vi "Old Mixed Mode Widget.vi"() -> ()   [LabVIEW 2009]
uses:
  lib/Data Access Objects/Metadata/LBCB Filter.ctl
  lib/Apps/App Parameters Actions.ctl
  lib/MixedMode/Mixed Mode Command Action.ctl
  lib/MixedMode/Target Data.ctl
  lib/MixedMode/Ramp Time Tuple.ctl
  lib/MixedMode/Messages/Mixed Mode Command.ctl
  lib/MixedMode/Mixed Mode Cartesian Data.ctl
  lib/MixedMode/Mixed Mode Covergance Status.ctl
  lib/MixedMode/Mixed Mode States.ctl
  lib/MixedMode/Messages/Mixed Mode Status.ctl
  lib/Launcher/NoPanelAppTypes.ctl
  lib/Launcher/Launcher Actions.ctl
  lib/MixedMode/Widget/Accepted or Declined.ctl
  lib/NTCP Client/NTCP Msg Types.ctl
  NTCP library/NTCP Commands.ctl
  NTCP library/NTCP Message.ctl
  lib/NTCP Client/NTCP States.ctl
  lib/NTCP Client/Control Point Suffix.ctl
  lib/MixedMode/Widget/Mixed Mode Widget Requests.ctl
  lib/MixedMode/Widget/MM Widget Parameter Changes.ctl
  lib/MixedMode/Widget/Step DAO Actions.ctl
  lib/MixedMode/Widget/Target.ctl
  NTCP library/Payload.ctl
  lib/MixedMode/Widget/Mixed Mode Widget State.ctl
  lib/MixedMode/Widget/NTCP MM Requests.ctl
  lib/Apps/App Status Actions.ctl
  lib/Data Access Objects/Metadata/LBCB Space.ctl
  lib/Global Data/Cartesian Measurment Actions.ctl
  lib/Data Access Objects/Metadata/LBCB Number.ctl
  lib/Global Data/Name Actions.ctl
  lib/Apps/AppStates.ctl
  lib/Control Loop/Parameter Change States.ctl
  lib/Control Loop/Parameters Changes.ctl
  lib/Apps/GUI Control.ctl
  lib/Data Access Objects/Metadata/Persistant DAO Actions.ctl
  lib/MixedMode/Widget/Mixed Mode State Display.ctl
  lib/MixedMode/Widget/Target Pattern.ctl
panel:
  in  "Cartesian Type":bool caption="CartesianType"
  out "NTCP MM Requests":T1
  in  "Connect Server Flag":bool
  out "Force Limit":bool caption="Force"
  out "Displacement Limit":bool caption="Displacement"
  out "Messages":string
  out "Mixed Mode Status":T2={"LBCB Target"=[], "MixedModeStates"=enum."Idle", "LBCB Convergence"=[], "LBCB Measurements"=[]}
  in  "App Running":bool
  out "Mixed Mode Widget Actions":T8
  out "Mixed Mode Widget Requests":T9
  in  "Stop":bool
  out "Mixed Mode Command":T11
  in  "Cartesian Type Button":bool caption="CartesianType"
  in  "Channel Data Tables":T14(tab)
  out "Cartesian Space Labels L1":string[](array[string])=["Commands (in/rad)", "Displacements (in/rad)", "Forces (lbs/lb*in)"]
  out "Cartesian Labels L1":string[](array[string])=["X", "Y", "Z", "Rx", "Ry", "Rz"]
  out "LBCB 1 Cartesian Space":dbl[][](array[numeric]) caption="LBCB 1"
  out "LBCB 2 Cartesian Space":dbl[][](array[numeric]) caption="LBCB 2"
  out "Cartesian Labels L2":string[](array[string])=["X", "Y", "Z", "Rx", "Ry", "Rz"]
  out "Cartesian Space Labels L2":string[](array[string])=["Commands (in/rad)", "Displacements (in/rad)", "Forces (lbs/lb*in)"]
  out "Actuator Space Labels L2":string[](array[string])=["Commands (in)", "Displacements (in)", "Forces (lbs)", "Integral"]
  out "Actuator Labels L2":string[](array[string])=["X1", "X2", "Y1", "Z1", "Z2", "Z3"]
  out "LBCB 2 Actuator Space":dbl[][](array[numeric]) caption="LBCB 2"
  out "LBCB 1 Actuator Space":dbl[][](array[numeric]) caption="LBCB 1"
  out "Actuator Labels L1":string[](array[string])=["X1", "X2", "Y1", "Z1", "Z2", "Z3"]
  out "Actuator Space Labels L1":string[](array[string])=["Commands (in)", "Displacements (in)", "Forces (lbs)", "Integral"]
  out "External Sensors":cluster{"Name":string, "Value":dbl}[](array[cluster])
  out "Test Statistics":cluster{"Steps":string, "Elapsed \nTime":dbl} {"Elapsed \nTime" format="%<%H:%M:%S>T"}
  in  "Mixed Mode Control Type":enum32{"Manual", "Input File", "NTCP"}(tab)
  in  "Target Pattern":T15
  in  "Apply Pattern":bool
  in  "Pause infile":bool
  in  "Run Infile":bool
  in  "Running":bool
  in  "Reset":bool
  in  "LBCB 1":path
  in  "Load File":bool
  in  "LBCB 2":path
  out "NTCP State":T16
  in  "Connect Server":bool
  in  "Control Point":string="MDL-00-01"
  out "Connected":bool
  in  "Execute":cluster{"Auto":bool, "Start":bool, "Stop":bool}
  in  "Propose":T17
  out "Mixed Mode State Display":T18
  out "Current Values":T19[](array[typedef])
  in  "Ramp Times":cluster{"Displacement":T13, "Force":T13}={"Displacement"={"Ramp"=5.0, "Stab"=4.0, "Hold"=5.0}, "Force"={"Ramp"=5.0, "Stab"=4.0, "Hold"=5.0}}
  in  "Targets":T19[](array[typedef])
  # "Limit\nFaults"
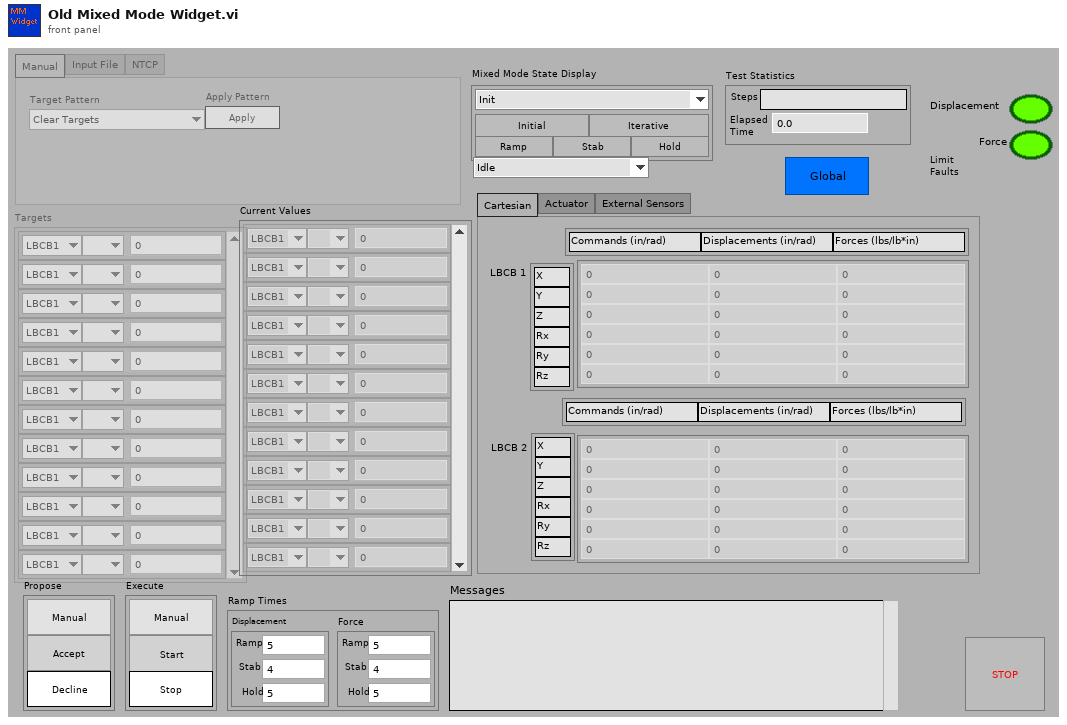
[diagram p1: front panel]
types:
  T1 = typedef "NTCP MM Requests.ctl" = cluster{"Execute Pending":bool, "Propose Pending":bool, "Connected":bool, "Reset":bool}
  T2 = typedef "Mixed Mode Status.ctl" = cluster{"LBCB Target":T3[], "MixedModeStates":T5, "LBCB Convergence":T6[], "LBCB Measurements":T7[]}
  T3 = typedef "Target Data.ctl" = cluster{"Displacements":dbl[], "Command Type":enum16{"<None>", "Displacement", "Force"}[], "Forces":dbl[], "Space":T4}
  T4 = typedef "LBCB Space.ctl" = enum16{"Actuator", "Cartesian"}
  T5 = typedef "Mixed Mode States.ctl" = enum16{"Init", "Wait For DAQ", "Idle", "Start Initial Position", "Initial Position", "Start Initial Ramp", "Run Initial Ramp", "Start Iterative Stage", "Convergence Check", "Update Stiffness Jacobian", "Update Command", "Start Iterative Ramp", "Run Iterative Ramp", "Start Iterative Stabilize", "Iterative Stabilize", "Start Iterative Holding", "Iterative Holding", "Start Stabilize", "Stabilize", "Start Hold", "Holding", "Done", "Aborting", "Exit", "Nop"}
  T6 = typedef "Mixed Mode Covergance Status.ctl" = cluster{"IsConverged":bool[], "Force Errors":dbl[], "MaxForceDiffIndex":i32}
  T7 = typedef "Mixed Mode Cartesian Data.ctl" = cluster{"Displacements":dbl[], "Forces":dbl[]}
  T8 = typedef "Mixed Mode Widget State.ctl" = enum16{"Idle", "Auto Start", "Wait for Start", "Start", "Wait for Hold", "Waiting for Done", "Step Completed", "Limit Fault", "Stop", "Abort", "Clear Targets", "Reset", "Steps Loaded", "Paused", "Steps Available", "Load Step", "Connected", "Disconnecting", "Wait for Proposal", "Auto Accept", "Wait for Accept", "Accept", "Decline", "Wait for Execute", "Unknown", "Exit"}
  T9 = typedef "Mixed Mode Widget Requests.ctl" = cluster{"Start Requested":bool, "Targets Updated":bool, "Targets Cleared":bool, "Stop Requested":bool, "Auto-Start Enabled":bool, "Auto-Accept Enabled":bool, "Accepted or Declined":T10, "Running":bool, "File Loaded":bool, "Reset":bool, "Exit Requested":bool}
  T10 = typedef "Accepted or Declined.ctl" = enum16{"No Decision Yet", "Accepted", "Declined"}
  T11 = typedef "Mixed Mode Command.ctl" = cluster{"Command":T12, "Ramp Times":cluster{"Initial":T13, "Iterative":T13}, "LBCB1":T3, "LBCB2":T3}
  T12 = typedef "Mixed Mode Command Action.ctl" = enum16{"Start Command", "Stop", "Exit", "No Op", "Start Acquisition", "Measure Initial Position"}
  T13 = typedef "Ramp Time Tuple.ctl" = cluster{"Ramp":dbl, "Stab":dbl, "Hold":dbl}
  T14 = enum32{"Cartesian", "Actuator", "External Sensors"}
  T15 = typedef "Target Pattern.ctl" = enum16{"Clear Targets", "Reset Targets to Zero", "Displacements Only", "Rotations Only", "Displacements & Rotations"}
  T16 = typedef "NTCP States.ctl" = enum16{"Init", "Disconnected", "Start Server", "Connect to Server", "Listening", "Parse Message", "Proposed", "Execute", "Get Control Point", "Shutdown Server"}
  T17 = cluster{"Auto":bool, "Accept":bool, "Decline":bool}
  T18 = typedef "Mixed Mode State Display.ctl" = cluster{"MixedModeStates":T5, "Initial":bool, "Iterative":bool, "Ramp":bool, "Stab":bool, "Hold":bool}
  T19 = typedef "Target.ctl" = cluster{"LBCB Number":T20, "DOF Vectors":enum16{" ", "Dx", "Dy", "Dz", "Rx", "Ry", "Rz", "Fx", "Fy", "Fz", "Mx", "My", "Mz"}, "Amount":dbl}
  T20 = typedef "LBCB Number.ctl" = enum16{"LBCB1", "LBCB2"}
  T21 = typedef "GUI Control.ctl" = cluster{"Command":T22, "LBCB Number":enum16{"LBCB1", "LBCB2"}}
  T22 = typedef "MM Widget Parameter Changes.ctl" = enum16{"Start", "Stop All", "Cartesian Type Changed", "Control Enabled", "Control Disabled"}
  T23 = typedef "Parameters Changes.ctl" = cluster{"Change State":T24, "LBCB Number":T20}
  T24 = typedef "Parameter Change States.ctl" = enum16{"Mixed Mode", "Control Loop", "Limits", "Application", "Stiffness Jacobian", "Start DAQ", "Auto-Balancing", "Set Command", "Enable Control", "Disable Control", "Stop Application"}
  T25 = typedef "Name Actions.ctl" = enum16{"Init", "Get Names", "Get Index"}
  T26 = typedef "LBCB Filter.ctl" = enum16{"LBCB 1", "LBCB 2", "Both"}
  T27 = typedef "NTCP Message.ctl" = cluster{"NTCP commands":T28, "Transaction ID":string, "Control Point":string, "Payload":T29[]}
  T28 = typedef "NTCP Commands.ctl" = enum16{"propose", "execute", "cancel", "set-parameter", "get-parameter", "open-session", "close-session", "get-control-point", "Unknown", "stop"}
  T29 = typedef "Payload.ctl" = cluster{"Content":string, "Control Point Suffix":T30}
  T30 = typedef "Control Point Suffix.ctl" = enum16{"LBCB1", "LBCB2", "ExternalSensors"}
  T31 = typedef "Launcher Actions.ctl" = enum16{"Launch", "Stop All", "Stop", "Kill", "Running?", "Init"}
  T32 = typedef "NoPanelAppTypes.ctl" = enum16{"NTCP Socket", "Data Archiving", "DAQ Link", "Control Loops", "Autobalance Monitor", "Mixed Mode Monitor", "Cart Plot", "Act Plot", "Cmd Disp Diffs"}
  T33 = typedef "App Status Actions.ctl" = enum16{"Init", "Get Status", "Running", "Control", "Autobalanced", "Data Acquisition", "Set App State", "DAQ Started", "Set LBCB State", "Set All", "Set Cont Logging", "Set Step Logging", "Set MM Logging", "Set Volt Logging", "Set Cart Type", "Set DAQ Link", "Set NTCP Link"}
  T34 = typedef "Step DAO Actions.ctl" = enum16{"Init", "Set", "Get", "Reset Count"}
  T35 = typedef "App Status.ctl" = cluster{"Running":bool, "Controlling L2":bool, "Autobalance L2":bool, "Data Acquisition":bool, " App State":T36, "DAQ Started":bool, "LBCB 1 State":T37, "LBCB 2 State":T37, "Controlling L1":bool, "Autobalance L1":bool, "Cartesian Type":bool, "Continuous Logging":bool, "Step Logging":bool, "Voltage Logging":bool, "Mixed Mode Logging":bool, "DAQ Link":bool, "NTCP Link ":bool}
  T36 = typedef "AppStates.ctl" = enum16{"Starting OM", "Initializing Displays", "Setting up Archiving", "Setting Up DAQ Channels", "Start DAQ", "DAQ Starting", "Controlling LBCBs", "Stopping OM"}
  T37 = typedef "Lbcb Control Loop States.ctl" = enum16{"Idle", "Start Selected", "Load Last Command", "Start Autobalancing", "Autobalancing", "Control Loop Initialized", "Control Enabled"}
  T38 = typedef "App Parameters Actions.ctl" = enum16{"Init", "Get", "Set"}
  T39 = typedef "Persistant DAO Actions.ctl" = enum16{"Init", "Get", "Set", "Load", "Save"}
  T40 = typedef "App Parameters.ctl" = cluster{"Monitor Loop":T41, "Ramp Time":T41, "Log Loop":T41, "TCP to DAQ":T41, "Logging Directory":path, "Log File Size (MBytes)":i64, "Volt Logging Loop":T41}
  T41 = typedef "Timing Parameters.ctl" = cluster{"Interval":dbl, "Rate ":dbl}
  T42 = typedef "Ramp Time Input.ctl" = cluster{"Directional":T43, "Iterative":T43}
  T43 = typedef "Ramp Control.ctl" = cluster{"Ramp":dbl, "Stabilize":dbl, "Hold":dbl}
  T44 = typedef "Mixed Mode Widget Button States.ctl" = cluster{"Auto-Start Enabled":bool, "Auto-Accept Enabled":bool, "Exit Requested":bool, "Mixed Mode Control Type":T45, "Input File Loaded":bool, "Input File Running":bool}
  T45 = typedef "Mixed Mode Control Type.ctl" = enum32{"Manual", "Input File", "NTCP"}
  T46 = typedef "Widget Changed.ctl" = cluster{"Running Changed":bool, "Apply Pattern Changed":bool, "Propose Changed":bool, "Execute Changed":bool, "Widget Requests Changed":bool}
  T47 = typedef "NTCP Msg Types.ctl" = enum16{"Control Point", "Step Done", "Propose Accepted", "Propose Not Accepted", "Propose Declined", "Propose Response", "Execute Done"}
  T48 = typedef "Cartesian Measurment Actions.ctl" = enum16{"Set Data", "Get", "Init", "Set Offsets"}
  T49 = typedef "Cartesian Data Type.ctl" = cluster{"Displacements":dbl[], "Forces":dbl[], "Displacement Commands":dbl[]}
  T50 = typedef "Propose Command.ctl" = cluster{"Control Type":i32[], "Value":dbl[]}
  T51 = typedef "Mixed Mode Blinkies.ctl" = cluster{"Blink Accept":bool, "Blink Start":bool, "Targets Updated":bool, "Disconnect":bool}
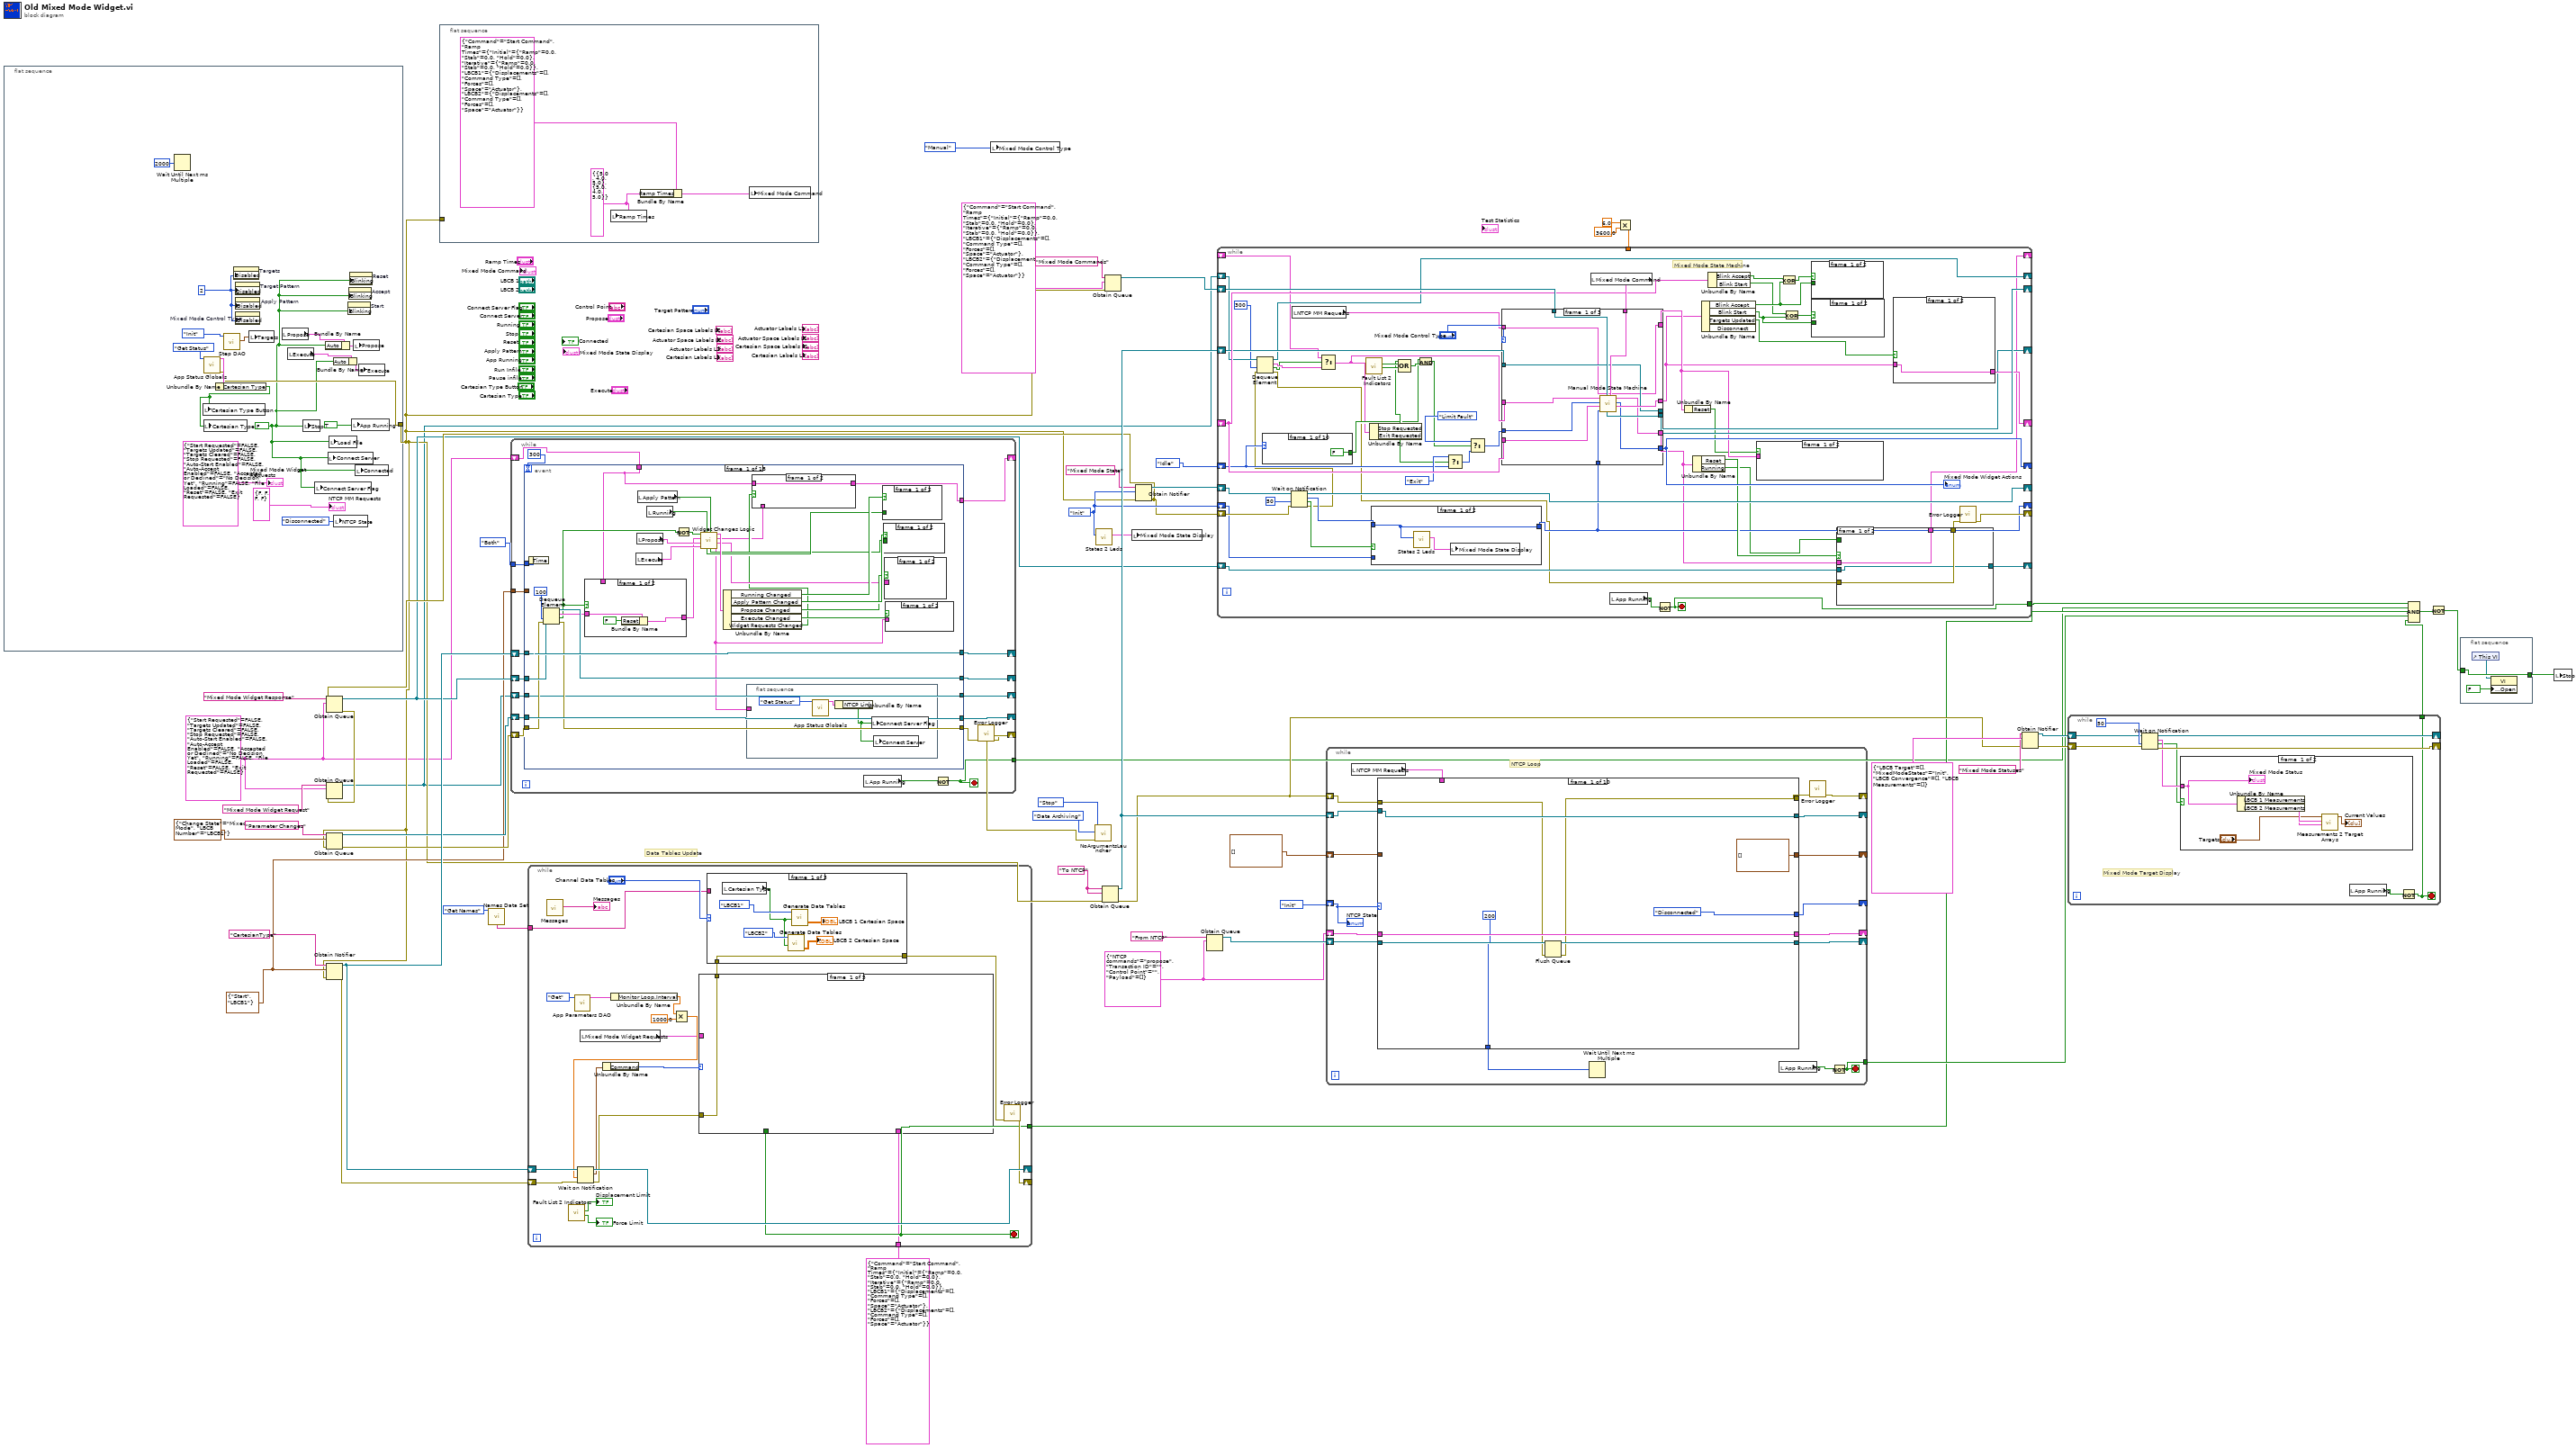
[diagram p0: block diagram]
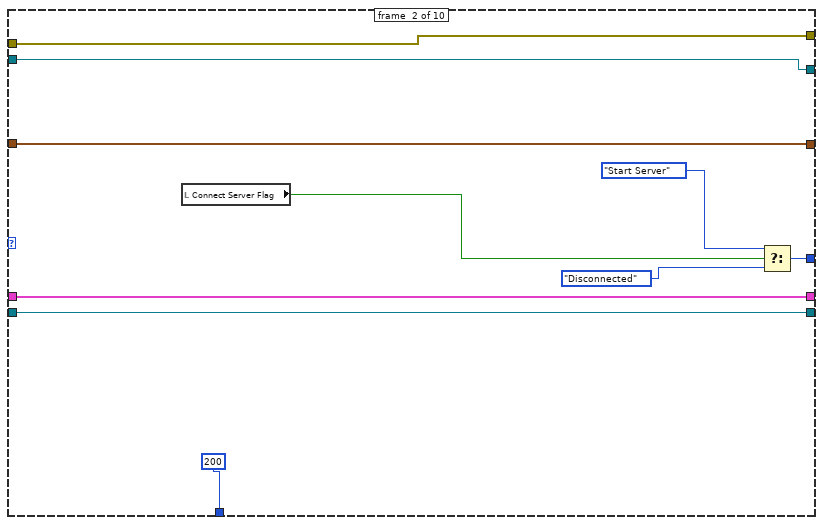
[diagram p3: hidden frame]
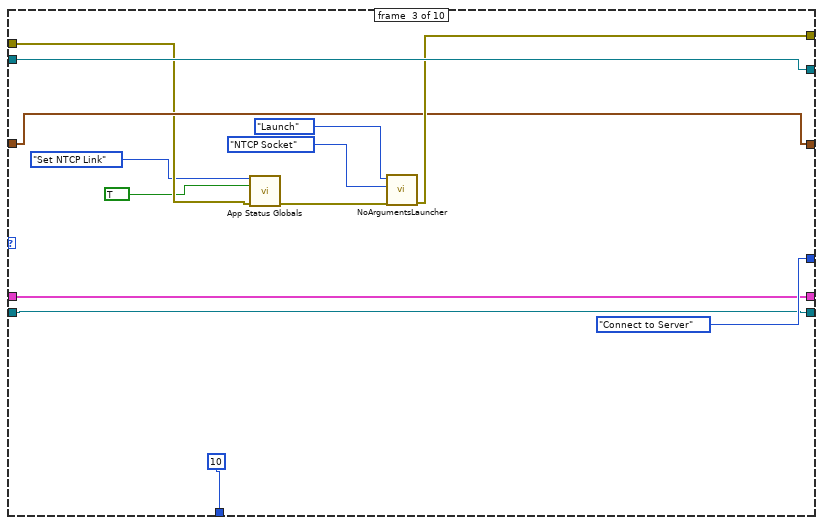
[diagram p4: hidden frame]
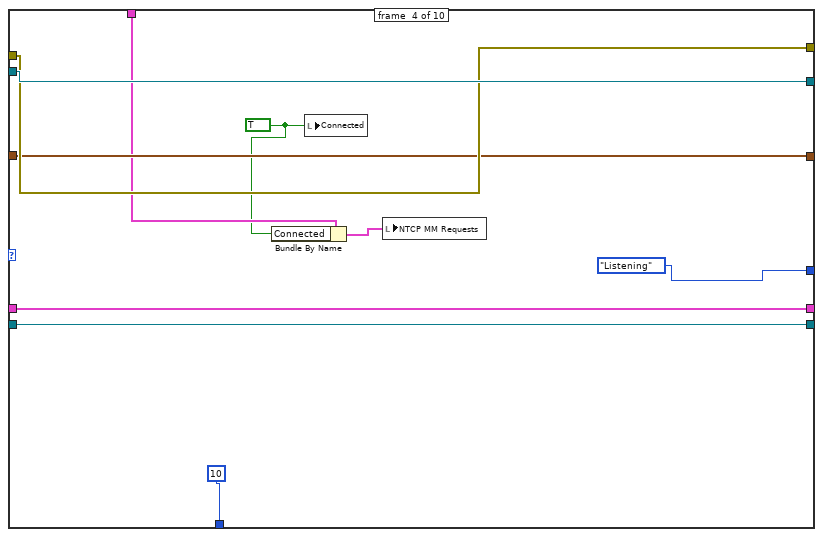
[diagram p5: hidden frame]
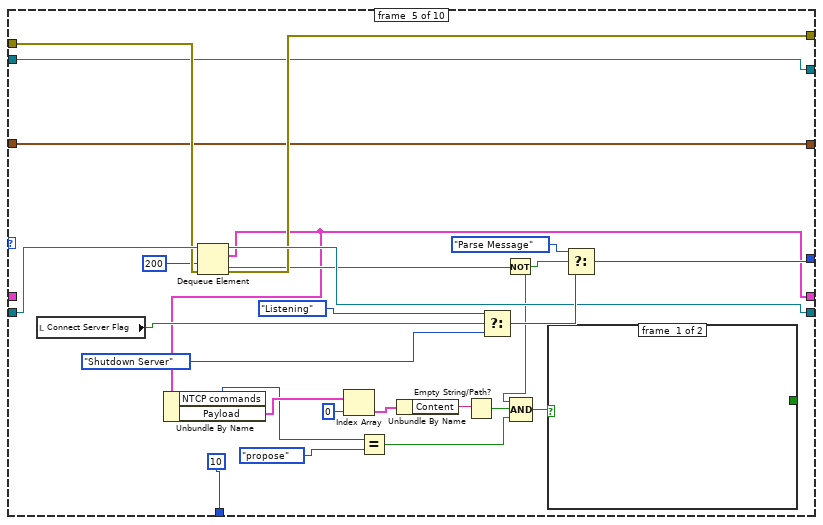
[diagram p6: hidden frame]
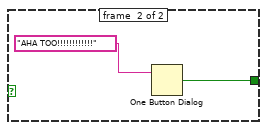
[diagram p7: hidden frame]
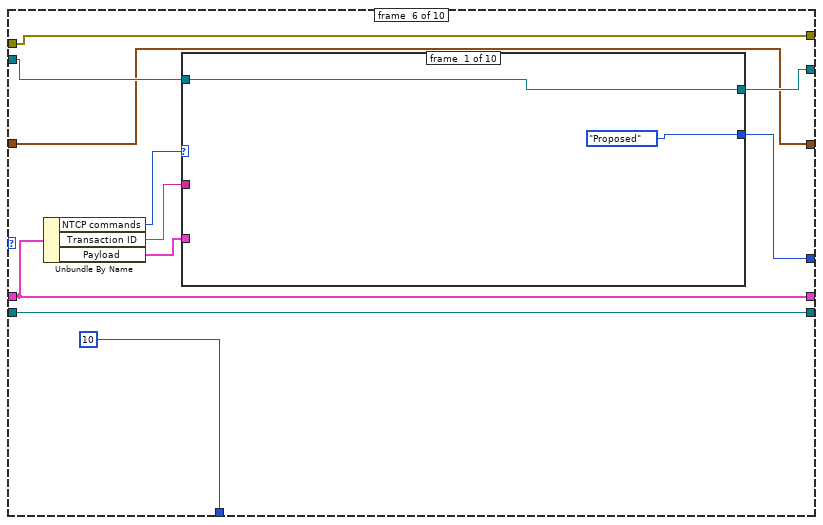
[diagram p8: hidden frame]
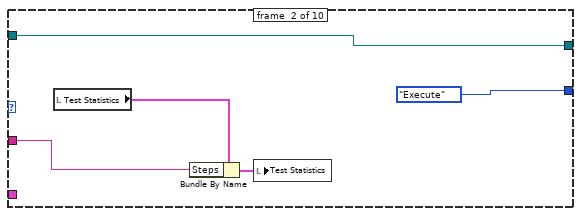
[diagram p9: hidden frame]
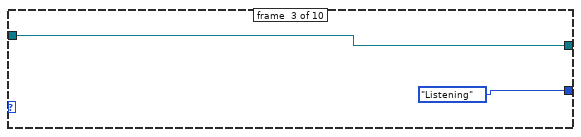
[diagram p10: hidden frame]
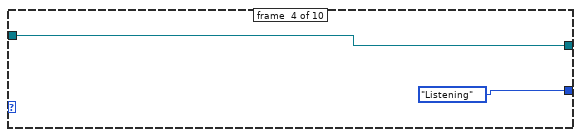
[diagram p11: hidden frame]
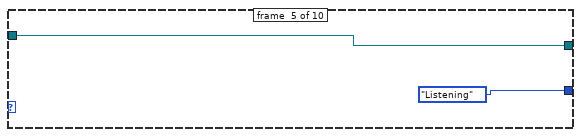
[diagram p12: hidden frame]
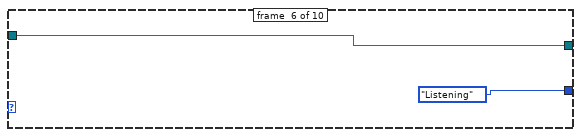
[diagram p13: hidden frame]
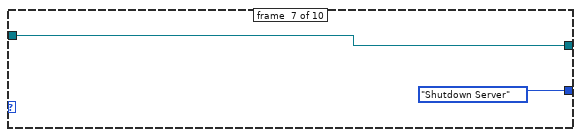
[diagram p14: hidden frame]
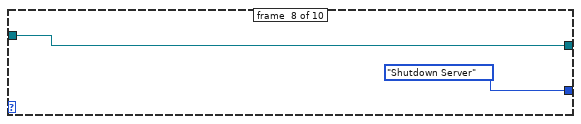
[diagram p15: hidden frame]
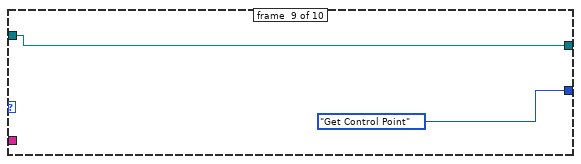
[diagram p16: hidden frame]
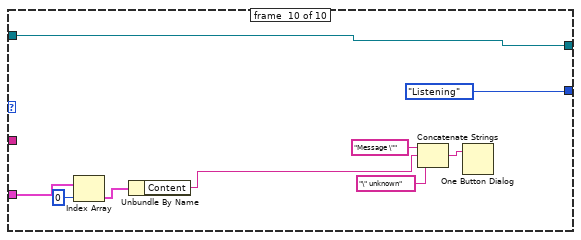
[diagram p17: hidden frame]
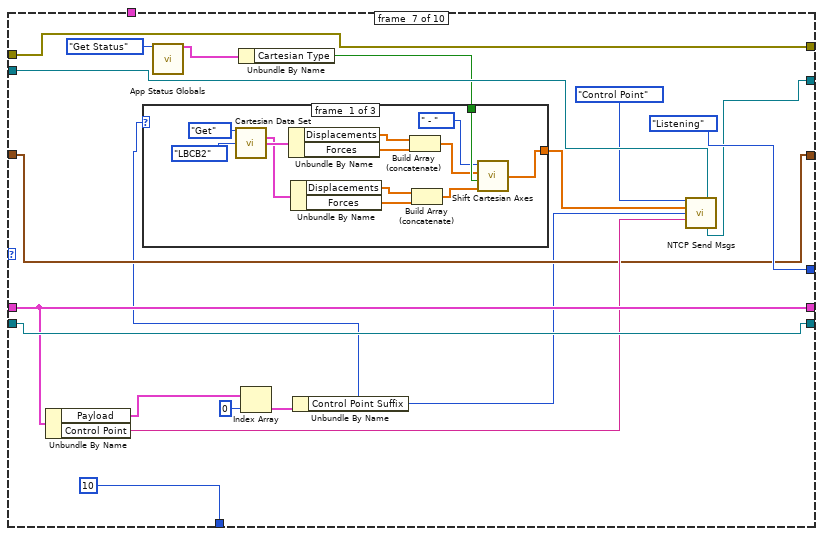
[diagram p18: hidden frame]
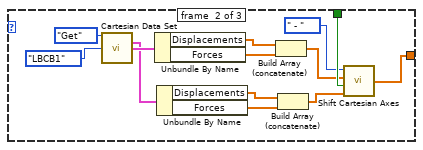
[diagram p19: hidden frame]
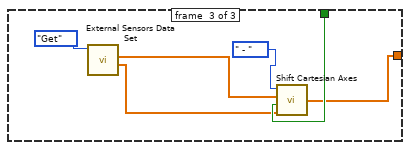
[diagram p20: hidden frame]
diagram:
  w17 = T21 {"Command"=enum."Start", "LBCB Number"=enum."LBCB1"} ("GUI Control")
  w5 = T9 {"Start Requested"=FALSE, "Targets Updated"=FALSE, "Targets Cleared"=FALSE, "Stop Requested"=FALSE, "Auto-Start Enabled"=FALSE, "Auto-Accept Enabled"=FALSE, "Accepted or Declined"=enum."No Decision Yet", "Running"=FALSE, "File Loaded"=FALSE, "Reset"=FALSE, "Exit Requested"=FALSE} ("Mixed Mode Widget Approval")
  w21 = Mixed_Mode_States."Init" ("MixedModeStates")
  w45 = T27 {"NTCP commands"=enum."propose", "Transaction ID"="", "Control Point"="", "Payload"=[]} ("NTCP Message")
  w2 = "To NTCP" ("name (unnamed)")
  # "Data Tables Update"
  n1 = flat-sequence {
    tunnel: [w71] -> w10
    frame #0 {
      w59 = u8 2 ("Disabled")
      w56 = FALSE ("Exit")
      n2 = Wait Until Next ms Multiple(millisecond multiple=u32 2000) -> ()  [unwired: 1 out]
      n3 = call "App Status Globals.vi"("App Status Actions"=App_Status_Actions."Get Status") -> ("App Status Out"=w72:T35, "error out"=w71:errorcluster)  [unwired: 5 in, 8 out]
      n4 = Unbundle By Name(w72) -> ("Cartesian Type"=w57:bool)
      n5 = local write "Cartesian Type Button"(w57) -> ()
      n6 = local write "Cartesian Type"(w57) -> ()
      n7 = call "Step DAO.vi"("Step DAO Actions"=Step_DAO_Actions."Init") -> ("Step Out"=w69:T19[])  [unwired: 3 in, 7 out]
      n8 = property on="Targets" class="Arr (strict)"("Disabled"=w59) -> ()  [unwired: 2 in, 2 out]
      n9 = property on="Target Pattern" class="Enum (strict)"("Disabled"=w59) -> ()  [unwired: 2 in, 2 out]
      n10 = property on="Apply Pattern" class="Bool (strict)"("Disabled"=w59) -> ()  [unwired: 2 in, 2 out]
      n11 = property on="Mixed Mode Control Type" class="TabCtl (strict)"("Disabled"=w59) -> ()  [unwired: 2 in, 2 out]
      n12 = local write "Targets"(w69) -> ()
      n13 = local read "Propose"() -> (w64:T17)
      n14 = local read "Execute"() -> (w62:cluster{"Auto":bool, "Start":bool, "Stop":bool})
      n15 = local write "Stop"(w56) -> ()
      n16 = local write "Connect Server Flag"(w56) -> ()
      n17 = Bundle By Name(cluster=w64, "Auto"=w56) -> (w65:T17)
      n18 = local write "Connect Server"(w56) -> ()
      n19 = local write "Load File"(w56) -> ()
      n20 = Bundle By Name(cluster=w62, "Auto"=w56) -> (w63:cluster{"Auto":bool, "Start":bool, "Stop":bool})
      n21 = local write "NTCP State"(NTCP_States."Disconnected" ("NTCP State")) -> ()
      n22 = property on="Start" class="Bool (strict)"("Blinking"=w56) -> ()  [unwired: 2 in, 2 out]
      n23 = property on="Accept" class="Bool (strict)"("Blinking"=w56) -> ()  [unwired: 2 in, 2 out]
      n24 = property on="Reset" class="Bool"("Blinking"=w56) -> ()  [unwired: 2 in, 2 out]
      n25 = local write "App Running"(TRUE) -> ()
      n26 = local write "Propose"(w65) -> ()
      n27 = local write "Connected"(w56) -> ()
      n28 = local write "Execute"(w63) -> ()
      "Mixed Mode Widget Requests" <- T9 {"Start Requested"=FALSE, "Targets Updated"=FALSE, "Targets Cleared"=FALSE, "Stop Requested"=FALSE, "Auto-Start Enabled"=FALSE, "Auto-Accept Enabled"=FALSE, "Accepted or Declined"=enum."No Decision Yet", "Running"=FALSE, "File Loaded"=FALSE, "Reset"=FALSE, "Exit Requested"=FALSE} ("Mixed Mode Widget Requests")
      "NTCP MM Requests" <- T1 {"Execute Pending"=FALSE, "Propose Pending"=FALSE, "Connected"=FALSE, "Reset"=FALSE} ("NTCP MM Requests")
    }
  }
  n29 = Obtain Queue(name (unnamed)="Parameter Changes", element data type=T23 {"Change State"=enum."Mixed Mode", "LBCB Number"=enum."LBCB1"} ("Parameter Changes"), error in (no error)=w10) -> (queue out=w28:refnum<queue>, error out=w29:errorcluster)  [unwired: 2 in, 1 out]
  n30 = Obtain Notifier(name (unnamed)="CartesianType", notification data type=w17, error in (no error)=w10) -> (notifier out=w48:refnum<notifier>, error out=w39:errorcluster)  [unwired: 1 in, 1 out]
  n31 = flat-sequence {
    tunnel: w10 -> [_]
    frame #0 {
      w73 = cluster{"Initial":T13, "Iterative":T13} {"Initial"={"Ramp"=5.0, "Stab"=4.0, "Hold"=5.0}, "Iterative"={"Ramp"=5.0, "Stab"=4.0, "Hold"=5.0}} ("Ramp Times")
      n32 = local write "Ramp Times"(w73) -> ()
      n33 = Bundle By Name(cluster=T11 {"Command"=enum."Start Command", "Ramp Times"={"Initial"={"Ramp"=0.0, "Stab"=0.0, "Hold"=0.0}, "Iterative"={"Ramp"=0.0, "Stab"=0.0, "Hold"=0.0}}, "LBCB1"={"Displacements"=[], "Command Type"=[], "Forces"=[], "Space"=enum."Actuator"}, "LBCB2"={"Displacements"=[], "Command Type"=[], "Forces"=[], "Space"=enum."Actuator"}} ("Mixed Mode Command"), "Ramp Times"=w73) -> (w75:T11)
      n34 = local write "Mixed Mode Command"(w75) -> ()
    }
  }
  n35 = call "Names Data Set.vi"("Name Actions"=Name_Actions."Get Names") -> ("External Sensor Names"=w32:string[])  [unwired: 1 in, 13 out]
  n36 = while {
    shift-right: [w91] -> _
    shift-left: w48 -> [w92]
    shift-right: [w87] -> _
    shift-left: w39 -> [w88]
    tunnel: w32 -> [w82]
    tunnel: [w80] -> w13
    tunnel: T11 {"Command"=enum."Start Command", "Ramp Times"={"Initial"={"Ramp"=0.0, "Stab"=0.0, "Hold"=0.0}, "Iterative"={"Ramp"=0.0, "Stab"=0.0, "Hold"=0.0}}, "LBCB1"={"Displacements"=[], "Command Type"=[], "Forces"=[], "Space"=enum."Actuator"}, "LBCB2"={"Displacements"=[], "Command Type"=[], "Forces"=[], "Space"=enum."Actuator"}} ("Mixed Mode Command") -> [w79]
    stop <- w80 stop-if-true
    n37 = call "Messages.vi"() -> ("Messages"=→"Messages":string)  [unwired: 2 in, 9 out]
    n38 = call "Fault List 2 Indicators.vi"() -> ("Forces"=→"Force Limit":bool, "Displacement"=→"Displacement Limit":bool)  [unwired: 1 in, 9 out]
    n39 = call "App Parameters DAO.vi"("Actions"=App_Parameters_Actions."Get" ("App Parameter Actions")) -> ("Application Timing and Logging Out"=w95:T40)  [unwired: 3 in, 7 out]
    n40 = local read "Mixed Mode Widget Requests"() -> (w83:T9)
    n41 = Unbundle By Name(w95) -> ("Monitor Loop.Interval"=w94:dbl)
    n42 = Multiply(x=w94, y=1000.0) -> (x*y=w90:dbl)
    n43 = Wait on Notification(notifier=w92, timeout in ms (-1)=w90, error in (no error)=w88) -> (notifier out=w91:refnum<notifier>, notification=w89:T21, error out=w78:errorcluster)  [unwired: 2 out]
    n44 = Unbundle By Name(w89) -> ("Command"=w81:T22)
    n45 = case shown="\"Cartesian Type Changed\"" w81 {
      tunnel: [_ w101 _ _ _] -> w80
      tunnel: w83 -> [_ w102 _ _ _]
      tunnel: w79 -> [_ _ _ w115 _]
      tunnel: w78 -> [w98 w99 w104 w114 w120]
      tunnel: [w98 w99 w104 w114 w120] -> w77
      frame #0 {
      }
      frame #1 {
        w101 = TRUE ("Exit")
        n46 = Bundle By Name(cluster=w102, "Exit Requested"=w101) -> (w100:T9)
        n47 = Not(x=w101) -> (.not. x?=w103:bool)
        n48 = local write "App Running"(w103) -> ()
        n49 = local write "Mixed Mode Widget Requests"(w100) -> ()
      }
      frame #2 {
        n50 = call "App Status Globals.vi"("App Status Actions"=App_Status_Actions."Get Status") -> ("App Status Out"=w107:T35)  [unwired: 5 in, 9 out]
        n51 = Unbundle By Name(w107) -> ("Cartesian Type"=w105:bool)
        n52 = local write "Cartesian Type"(w105) -> ()
        n53 = case shown="False" w105 {
          frame #0 {
            n54 = local read "Targets"() -> (w110:T19[])
            n55 = call "Local2Global Target Values.vi"("Direction"=enum16{" +", " - "}." - ", "Target  Inputs"=w110) -> ("Target  Outputs"=w109:T19[])  [unwired: 9 in]
            n56 = local write "Targets"(w109) -> ()
          }
          frame #1 {
            n57 = local read "Targets"() -> (w113:T19[])
            n58 = call "Local2Global Target Values.vi"("Direction"=enum16{" +", " - "}." +", "Target  Inputs"=w113) -> ("Target  Outputs"=w112:T19[])  [unwired: 9 in]
            n59 = local write "Targets"(w112) -> ()
          }
        }
      }
      frame #3 {
        w119 = u8 0 ("Disabled")
        n60 = property on="Target Pattern" class="Enum (strict)"("Disabled"=w119) -> ()  [unwired: 2 in, 2 out]
        n61 = property on="Targets" class="Arr (strict)"("Disabled"=w119) -> ()  [unwired: 2 in, 2 out]
        n62 = property on="Apply Pattern" class="Bool (strict)"("Disabled"=w119) -> ()  [unwired: 2 in, 2 out]
        n63 = call "Default Ramp Time DAO.vi"("Ramp Time Actions"=Persistant_DAO_Actions."Get") -> ("Ramp Time Out"=w117:T42)  [unwired: 3 in, 11 out]
        n64 = property on="Mixed Mode Control Type" class="TabCtl (strict)"("Disabled"=w119) -> ()  [unwired: 2 in, 2 out]
        n65 = Bundle By Name(cluster=w115, "Ramp Times"=w117) -> (w116:T11)
        n66 = local write "Ramp Times"(w117) -> ()
        n67 = local write "Mixed Mode Command"(w116) -> ()
      }
      frame #4 {
        w121 = u8 2 ("Disabled")
        n68 = property on="Target Pattern" class="Enum (strict)"("Disabled"=w121) -> ()  [unwired: 2 in, 2 out]
        n69 = property on="Targets" class="Arr (strict)"("Disabled"=w121) -> ()  [unwired: 2 in, 2 out]
        n70 = property on="Apply Pattern" class="Bool (strict)"("Disabled"=w121) -> ()  [unwired: 2 in, 2 out]
        n71 = property on="Mixed Mode Control Type" class="TabCtl (strict)"("Disabled"=w121) -> ()  [unwired: 2 in, 2 out]
      }
    }
    n72 = case shown="\"External Sensors\"" "Channel Data Tables" {
      tunnel: w82 -> [_ _ w136]
      tunnel: w77 -> [w123 w128 w135]
      tunnel: [w123 w128 w135] -> w76
      frame #0 {
        n73 = local read "Cartesian Type"() -> (w122:bool)
        n74 = call "Generate Data Tables.vi"("LBCB Number"=LBCB_Number."LBCB2", "Cartesian Type"=w122) -> ("Cartesian Table"=→"LBCB 2 Cartesian Space":dbl[][])  [unwired: 1 in, 3 out]
        n75 = call "Generate Data Tables.vi"("LBCB Number"=LBCB_Number."LBCB1", "Cartesian Type"=w122) -> ("Cartesian Table"=→"LBCB 1 Cartesian Space":dbl[][])  [unwired: 1 in, 3 out]
      }
      frame #1 {
        w129 = FALSE ("Cartesian Type")
        # "Cartesian Type ignored\nbecause we are  using \nActuator Space"
        n76 = call "Generate Data Tables.vi"("LBCB Number"=LBCB_Number."LBCB1", "Cartesian Type"=w129) -> ("Actuator Table"=→"LBCB 1 Actuator Space":dbl[][])  [unwired: 1 in, 3 out]
        n77 = call "Generate Data Tables.vi"("LBCB Number"=LBCB_Number."LBCB2", "Cartesian Type"=w129) -> ("Actuator Table"=→"LBCB 2 Actuator Space":dbl[][])  [unwired: 1 in, 3 out]
      }
      frame #2 {
        n78 = local read "Cartesian Type"() -> (w134:bool)
        n79 = call "Generate External Sensors Table.vi"("External Sensor Names"=w136, "WithOffset"=w134) -> ("External Sensors"=→"External Sensors":cluster{"Name":string, "Value":dbl}[])  [unwired: 9 out]
      }
    }
    n80 = call "Error Logger.vi"("error in (no error)"=w76) -> ("error out"=w87:errorcluster)  [unwired: 1 in, 9 out]
  }
  n81 = local write "Mixed Mode Control Type"(enum32{"Manual", "Input File", "NTCP"}."Manual" ("Mixed Mode Control Type")) -> ()
  n82 = call "States 2 Leds.vi"("MixedModeStates"=w21) -> ("Mixed Mode State Display"=w20:T18)  [unwired: 10 out]
  n83 = Obtain Queue(name (unnamed)=w2, element data type=w2, error in (no error)=w10) -> (queue out=w44:refnum<queue>, error out=w22:errorcluster)  [unwired: 2 in, 1 out]
  n84 = Obtain Queue(name (unnamed)="Mixed Mode Commands", element data type=T11 {"Command"=enum."Start Command", "Ramp Times"={"Initial"={"Ramp"=0.0, "Stab"=0.0, "Hold"=0.0}, "Iterative"={"Ramp"=0.0, "Stab"=0.0, "Hold"=0.0}}, "LBCB1"={"Displacements"=[], "Command Type"=[], "Forces"=[], "Space"=enum."Actuator"}, "LBCB2"={"Displacements"=[], "Command Type"=[], "Forces"=[], "Space"=enum."Actuator"}} ("Mixed Mode Command"), error in (no error)=w10) -> (queue out=w40:refnum<queue>)  [unwired: 2 in, 2 out]
  n85 = local write "Mixed Mode State Display"(w20) -> ()
  n86 = Obtain Notifier(name (unnamed)="Mixed Mode State", notification data type=w21, error in (no error)=w10) -> (notifier out=w23:refnum<notifier>, error out=w19:errorcluster)  [unwired: 1 in, 1 out]
  n87 = Obtain Queue(name (unnamed)="Mixed Mode Widget Response", element data type=w5, error in (no error)=w19) -> (queue out=w18:refnum<queue>, error out=w7:errorcluster)  [unwired: 2 in, 1 out]
  n88 = Obtain Queue(name (unnamed)="Mixed Mode Widget Request", element data type=w5, error in (no error)=w7) -> (queue out=w6:refnum<queue>)  [unwired: 2 in, 2 out]
  n89 = while {
    shift-right: [w153] -> w33
    shift-left: w29 -> [w155]
    shift-right: [w150] -> _
    shift-left: w48 -> [w151]
    tunnel: LBCB_Filter."Both" ("LBCB Filter") -> [w149]
    shift-right: [w147] -> _
    shift-left: w28 -> [w148]
    shift-right: [w144] -> _
    shift-left: w18 -> [w145]
    tunnel: w17 -> [w143]
    tunnel: [w142] -> w12
    shift-right: [w138] -> _
    shift-left: w6 -> [w139]
    shift-right: [w141] -> _
    shift-left: w5 -> [w140]
    stop <- w142 stop-if-true
    n90 = event shown="[10] \"Load File\": Value Change" {
      selector: _ -> [_ _ _ _ _ _ _ _ _ _ _ _ _ _ _ _ _ _]
      dyn-events: _ -> [_ _ _ _ _ _ _ _ _ _ _ _ _ _ _ _ _ _]
      timeout: 300 -> [_ _ _ _ _ _ _ _ _ _ _ _ _ _ _ _ _ _]
      tunnel: w155 -> [w181 w203 w228 w256 w269 w283 w313 w329 w339 w359 w373 w398 w408 w419 w426 w443 w471 w476]
      tunnel: [w180 w198 w225 w254 w269 w281 w312 w330 w333 w358 w372 w398 w407 w418 w425 w441 w471 w475] -> w154
      tunnel: w151 -> [w184 w209 w235 w263 w268 w284 w318 w328 w344 w365 w375 w397 w412 w422 w439 w453 w472 w481]
      tunnel: [w184 w209 w235 w263 w268 w282 w318 w327 w344 w365 w375 w397 w412 w422 w439 w453 w472 w481] -> w150
      tunnel: w140 -> [w158 w208 w234 w262 w265 w280 w317 w320 w343 w364 w374 w392 w413 w423 w432 w452 w467 w483]
      tunnel: w149 -> [_ _ _ _ _ _ _ _ _ _ _ _ _ _ _ _ _ _]
      tunnel: w148 -> [w183 w206 w231 w260 w267 w278 w315 w325 w341 w361 w370 w395 w411 w421 w431 w451 w470 w480]
      tunnel: [w183 w206 w231 w260 w267 w278 w315 w325 w341 w361 w370 w395 w411 w421 w431 w451 w470 w480] -> w147
      tunnel: w145 -> [w182 w205 w230 w259 w266 w277 w314 w324 w340 w360 w369 w394 w409 w420 w429 w450 w469 w479]
      tunnel: [w178 w205 w230 w259 w266 w277 w314 w324 w340 w360 w369 w394 w409 w420 w429 w450 w469 w479] -> w144
      tunnel: w143 -> [_ _ _ _ _ w276 _ w323 _ _ _ _ _ _ _ _ _ _]
      tunnel: [w159 w202 w229 w258 w265 w275 w309 w320 w337 w355 w367 w392 w404 w415 w428 w444 w467 w477] -> w141
      tunnel: w139 -> [w157 w201 w227 w257 w264 w274 w311 w319 w336 w357 w368 w393 w406 w417 w427 w442 w468 w478]
      tunnel: [w157 w199 w226 w255 w264 w273 w310 w319 w334 w356 w366 w393 w405 w416 w424 w440 w468 w474] -> w138
      event #0 {
        n91 = event-data() -> ()  [unwired: 2 out]
        n92 = Dequeue Element(queue=w182, timeout in ms (-1)=100, error in (no error)=w181) -> (queue out=w178:refnum<queue>, element=w177:T9, timed out?=w173:bool, error out=w180:errorcluster)
        n93 = case shown="True" w173 {
          tunnel: w177 -> [w196 _]
          tunnel: w158 -> [_ w197]
          tunnel: [w195 w197] -> w174
          frame #0 {
            n94 = Bundle By Name(cluster=w196, "Reset"=FALSE) -> (w195:T9)
          }
          frame #1 {
          }
        }
        n95 = local read "Execute"() -> (w176:cluster{"Auto":bool, "Start":bool, "Stop":bool})
        n96 = local read "Propose"() -> (w175:T17)
        n97 = local read "Apply Pattern"() -> (w170:bool)
        n98 = local read "Running"() -> (w171:bool)
        n99 = Not(x=w173) -> (.not. x?=w172:bool)
        n100 = call "Widget Changes Logic.vi"("Apply Pattern In"=w170, "Running In"=w171, "Execute In"=w176, "Propose In"=w175, "Mixed Mode Widget Requests"=w174, "Mixed Mode Response Received"=w172) -> ("Execute Out"=w156:cluster{"Auto":bool, "Start":bool, "Stop":bool}, "Propose Out"=w163:T17, "Mixed Mode Widget Requests Out"=w160:T44, "Widget Changed"=w169:T46, "Apply Pattern Out"=w165:bool, "Running Out"=w167:bool)
        n101 = Unbundle By Name(w169) -> ("Running Changed"=w168:bool, "Apply Pattern Changed"=w166:bool, "Propose Changed"=w164:bool, "Execute Changed"=w162:bool, "Widget Requests Changed"=w161:bool)
        n102 = flat-sequence {
          tunnel: w156 -> [_]
          frame #0 {
            n103 = call "App Status Globals.vi"("App Status Actions"=App_Status_Actions."Get Status") -> ("App Status Out"=w186:T35)  [unwired: 13 in, 1 out]
            n104 = Unbundle By Name(w186) -> ("NTCP Link"=w185:bool)
            n105 = local write "Connect Server Flag"(w185) -> ()
            n106 = local write "Connect Server"(w185) -> ()
          }
        }
        n107 = case shown="False" w161 {
          tunnel: w160 -> [_ w189]
          tunnel: [w188 w189] -> w159
          tunnel: w158 -> [w188 _]
          frame #0 {
          }
          frame #1 {
          }
        }
        n108 = case shown="False" w168 {
          tunnel: w167 -> [_ w193]
          frame #0 {
          }
          frame #1 {
            n109 = local write "Running"(w193) -> ()
          }
        }
        n110 = case shown="False" w166 {
          tunnel: w165 -> [_ w192]
          frame #0 {
          }
          frame #1 {
            n111 = local write "Apply Pattern"(w192) -> ()
          }
        }
        n112 = case shown="False" w164 {
          tunnel: w163 -> [_ w191]
          frame #0 {
          }
          frame #1 {
            n113 = local write "Propose"(w191) -> ()
          }
        }
        n114 = case shown="True" w162 {
          tunnel: w156 -> [_ w190]
          frame #0 {
          }
          frame #1 {
            n115 = local write "Execute"(w190) -> ()
          }
        }
      }
      event #1 {
        n116 = event-data() -> ()  [unwired: 2 out]
        n117 = property on="Start" class="Bool (strict)"(error in=w203) -> (error out=w200:errorcluster, "Blinking"=w204:bool)  [unwired: 1 in, 1 out]
        n118 = case shown="False" w204 {
          tunnel: w208 -> [w210 w219]
          tunnel: [w210 w215] -> w202
          tunnel: w201 -> [w212 w217]
          tunnel: w200 -> [w211 w216]
          tunnel: [w212 w214] -> w199
          tunnel: [w211 w213] -> w198
          frame #0 {
          }
          frame #1 {
            n119 = Bundle By Name(cluster=w219, "Start Requested"=TRUE) -> (w215:T9)
            n120 = Enqueue Element(queue=w217, element=w215, error in (no error)=w216) -> (queue out=w214:refnum<queue>, error out=w213:errorcluster)  [unwired: 2 out]
          }
        }
        n121 = event-data("Discard?"=TRUE) -> ()  [unwired: 1 in, 1 out]
      }
      event #2 {
        n122 = event-data() -> ("NewVal"=w224:T19[])  [unwired: 1 out]
        n123 = local read "Cartesian Type"() -> (w222:bool)
        n124 = case shown="False" w222 {
          tunnel: w224 -> [w240 w243]
          tunnel: [w240 w242] -> w223
          frame #0 {
          }
          frame #1 {
            n125 = call "Local2Global Target Values.vi"("Direction"=enum16{" +", " - "}." +", "Target  Inputs"=w243) -> ("Target  Outputs"=w242:T19[])  [unwired: 9 in]
          }
        }
        n126 = call "Step DAO.vi"("Step In"=w223, "Step DAO Actions"=Step_DAO_Actions."Set") -> ("Step Out"=w220:T19[], "Duplicates found"=w232:bool)  [unwired: 2 in, 6 out]
        n127 = case shown="False" w232 {
          tunnel: w234 -> [w250 w251]
          tunnel: [w246 w251] -> w229
          tunnel: w228 -> [w247 w253]
          tunnel: w227 -> [w248 w252]
          tunnel: [w245 w252] -> w226
          tunnel: [w244 w253] -> w225
          frame #0 {
            n128 = Bundle By Name(cluster=w250, "Targets Updated"=TRUE) -> (w246:T9)
            n129 = Enqueue Element(queue=w248, element=w246, error in (no error)=w247) -> (queue out=w245:refnum<queue>, error out=w244:errorcluster)  [unwired: 2 out]
          }
          frame #1 {
          }
        }
        n130 = case shown="False" w222 {
          tunnel: w220 -> [w236 w239]
          tunnel: [w236 w238] -> w221
          frame #0 {
          }
          frame #1 {
            n131 = call "Local2Global Target Values.vi"("Direction"=enum16{" +", " - "}." - ", "Target  Inputs"=w239) -> ("Target  Outputs"=w238:T19[])  [unwired: 9 in]
          }
        }
        n132 = local write "Targets"(w221) -> ()
      }
      event #3 {
        n133 = event-data() -> ("NewVal"=w261:bool)  [unwired: 1 out]
        n134 = Bundle By Name(cluster=w262, "Auto-Start Enabled"=w261) -> (w258:T9)
        n135 = Enqueue Element(queue=w257, element=w258, error in (no error)=w256) -> (queue out=w255:refnum<queue>, error out=w254:errorcluster)  [unwired: 2 out]
      }
      event #4 {
        n136 = event-data() -> ("NewVal"=w271:cluster{"Displacement":T13, "Force":T13})  [unwired: 1 out]
        n137 = local read "Mixed Mode Command"() -> (w272:T11)
        n138 = Bundle By Name(cluster=w272, "Ramp Times"=w271) -> (w270:T11)
        n139 = local write "Mixed Mode Command"(w270) -> ()
      }
      event #5 {
        n140 = event-data() -> ("NewVal"=w279:bool)  [unwired: 1 out]
        n141 = case shown="True" w279 {
          selector: w279 -> [_ w300]
          tunnel: w284 -> [w288 w304]
          tunnel: w283 -> [w287 w303]
          tunnel: [w288 w302] -> w282
          tunnel: [w287 w292] -> w281
          tunnel: w280 -> [w286 w301]
          tunnel: w276 -> [_ w294]
          tunnel: [w286 w289] -> w275
          tunnel: w274 -> [w285 w291]
          tunnel: [w285 w290] -> w273
          frame #0 {
          }
          frame #1 {
            n142 = Bundle By Name(cluster=w294, "Command"=MM_Widget_Parameter_Changes."Stop All" ("notification")) -> (w296:T21)
            n143 = Not(x=w300) -> (.not. x?=w298:bool)
            n144 = Send Notification(notification=w296, notifier=w304, error in (no error)=w303) -> (notifier out=w302:refnum<notifier>, error out=w293:errorcluster)
            n145 = Bundle By Name(cluster=w301, "Stop Requested"=w300) -> (w289:T9)
            n146 = local write "App Running"(w298) -> ()
            n147 = call "App Status Globals.vi"("App Status Actions"=App_Status_Actions."Running", "Status\nSetting"=w298) -> ("error out"=w306:errorcluster)  [unwired: 5 in, 8 out]
            n148 = Enqueue Element(queue=w291, element=w289, error in (no error)=w293) -> (queue out=w290:refnum<queue>, error out=w292:errorcluster)  [unwired: 2 out]
            n149 = call "App Status Globals.vi"("App Status Actions"=App_Status_Actions."Set App State", "App State"=AppStates."Stopping OM", "error in (no error)"=w306) -> ()  [unwired: 3 in, 10 out]
          }
        }
      }
      event #6 {
        w307 = FALSE ("Status\nSetting")
        n150 = event-data() -> ()  [unwired: 9 out]
        n151 = Bundle By Name(cluster=w317, "Stop Requested"=TRUE) -> (w309:T9)
        n152 = call "App Status Globals.vi"("App Status Actions"=App_Status_Actions."Set NTCP Link", "Status\nSetting"=w307) -> ()  [unwired: 12 in, 2 out]
        n153 = Enqueue Element(queue=w311, element=w309, error in (no error)=w313) -> (queue out=w310:refnum<queue>, error out=w312:errorcluster)  [unwired: 2 out]
        n154 = local write "Connect Server Flag"(w307) -> ()
        n155 = local write "Connect Server"(w307) -> ()
      }
      event #7 {
        n156 = event-data() -> ("NewVal"=w331:bool)  [unwired: 1 out]
        n157 = call "App Status Globals.vi"("App Status Actions"=App_Status_Actions."Set Cart Type", "Status\nSetting"=w331, "error in (no error)"=w329) -> ("error out"=w332:errorcluster)  [unwired: 3 in, 9 out]
        n158 = Bundle By Name(cluster=w323, "Command"=MM_Widget_Parameter_Changes."Cartesian Type Changed" ("notification")) -> (w321:T21)
        n159 = Send Notification(notification=w321, notifier=w328, error in (no error)=w332) -> (notifier out=w327:refnum<notifier>, error out=w330:errorcluster)
      }
      event #8 {
        n160 = event-data() -> ()  [unwired: 2 out]
        n161 = property on="Accept" class="Bool (strict)"(error in=w339) -> (error out=w335:errorcluster, "Blinking"=w338:bool)  [unwired: 1 in, 1 out]
        n162 = case shown="True" w338 {
          tunnel: w343 -> [w345 w354]
          tunnel: [w345 w350] -> w337
          tunnel: w336 -> [w346 w351]
          tunnel: w335 -> [w347 w352]
          tunnel: [w346 w349] -> w334
          tunnel: [w347 w348] -> w333
          frame #0 {
          }
          frame #1 {
            n163 = Bundle By Name(cluster=w354, "Accepted or Declined"=Accepted_or_Declined."Accepted") -> (w350:T9)
            n164 = Enqueue Element(queue=w351, element=w350, error in (no error)=w352) -> (queue out=w349:refnum<queue>, error out=w348:errorcluster)  [unwired: 2 out]
          }
        }
        n165 = event-data("Discard?"=TRUE) -> ()  [unwired: 1 in, 1 out]
      }
      event #9 {
        n166 = event-data() -> ()  [unwired: 9 out]
        n167 = Bundle By Name(cluster=w364, "Accepted or Declined"=Accepted_or_Declined."Declined") -> (w355:T9)
        n168 = Enqueue Element(queue=w357, element=w355, error in (no error)=w359) -> (queue out=w356:refnum<queue>, error out=w358:errorcluster)  [unwired: 2 out]
        n169 = event-data("Discard?"=TRUE) -> ()  [unwired: 1 in, 1 out]
      }
      event #10 {
        n170 = event-data() -> ("NewVal"=w371:bool)  [unwired: 1 out]
        n171 = case shown="True" w371 {
          tunnel: w374 -> [w377 w391]
          tunnel: w373 -> [w378 w390]
          tunnel: [w378 w382] -> w372
          tunnel: w368 -> [w376 w381]
          tunnel: [w377 w380] -> w367
          tunnel: [w376 w379] -> w366
          frame #0 {
          }
          frame #1 {
            n172 = local read "LBCB 2"() -> (w384:path)
            n173 = local read "LBCB 1"() -> (w385:path)
            n174 = call "Input File Step Iterator.vi"("error in (no error)"=w390, 9:w384, "LBCB Input Files"=w385, "Input File Step Actions"=enum16{"Load", "Next Step", "Reset"}."Load") -> ("error out"=w383:errorcluster)  [unwired: 7 out]
            n175 = Bundle By Name(cluster=w391, "File Loaded"=TRUE ("Targets Updated")) -> (w380:T9)
            n176 = local write "Load File"(FALSE ("Load File")) -> ()
            n177 = property on="Reset" class="Bool"("Disabled"=u8 0) -> ()  [unwired: 2 in, 2 out]
            n178 = Enqueue Element(queue=w381, element=w380, error in (no error)=w383) -> (queue out=w379:refnum<queue>, error out=w382:errorcluster)  [unwired: 2 out]
          }
        }
      }
      event #11 {
        n179 = event-data() -> ()  [unwired: 2 out]
        n180 = local read "Running"() -> (w396:bool)
        n181 = case shown="False" w396 {
          frame #0 {
            n182 = call "Input File Step Iterator.vi"("Input File Step Actions"=enum16{"Load", "Next Step", "Reset"}."Reset") -> ()  [unwired: 2 in, 9 out]
          }
          frame #1 {
          }
        }
      }
      event #12 {
        w401 = FALSE ("Auto")
        n183 = event-data() -> ()  [unwired: 3 out]
        n184 = local read "Execute"() -> (w402:cluster{"Auto":bool, "Start":bool, "Stop":bool})
        n185 = Bundle By Name(cluster=w402, "Auto"=w401) -> (w403:cluster{"Auto":bool, "Start":bool, "Stop":bool})
        n186 = local write "Execute"(w403) -> ()
        n187 = Bundle By Name(cluster=w413, "Running"=FALSE) -> (w410:T9)
        n188 = Bundle By Name(cluster=w410, "Auto-Start Enabled"=w401) -> (w404:T9)
        n189 = Enqueue Element(queue=w406, element=w404, error in (no error)=w408) -> (queue out=w405:refnum<queue>, error out=w407:errorcluster)  [unwired: 1 in, 1 out]
      }
      event #13 {
        n190 = event-data() -> ()  [unwired: 3 out]
        n191 = Bundle By Name(cluster=w423, "Running"=TRUE) -> (w415:T9)
        n192 = Enqueue Element(queue=w417, element=w415, error in (no error)=w419) -> (queue out=w416:refnum<queue>, error out=w418:errorcluster)  [unwired: 1 in, 1 out]
      }
      event #14 {
        w430 = FALSE
        n193 = event-data() -> ()  [unwired: 2 out]
        n194 = property on="Load File" class="Bool (strict)"("Disabled"=u8 0) -> ()  [unwired: 2 in, 2 out]
        n195 = local write "Targets"(T19[] [] ("Targets")) -> ()
        n196 = local read "Execute"() -> (w435:cluster{"Auto":bool, "Start":bool, "Stop":bool})
        n197 = Bundle By Name(cluster=w432, "Auto-Start Enabled"=w430, "Auto-Accept Enabled"=w430, "File Loaded"=w430, "Targets Updated"=w430) -> (w428:T9)
        n198 = local write "Running"(w430) -> ()
        n199 = local read "Propose"() -> (w436:T17)
        n200 = Bundle By Name(cluster=w435, "Auto"=w430) -> (w437:cluster{"Auto":bool, "Start":bool, "Stop":bool})
        n201 = Bundle By Name(cluster=w436, "Auto"=w430) -> (w438:T17)
        n202 = local write "Execute"(w437) -> ()
        n203 = local write "Propose"(w438) -> ()
        n204 = Enqueue Element(queue=w427, element=w428, error in (no error)=w426) -> (queue out=w424:refnum<queue>, error out=w425:errorcluster)  [unwired: 2 out]
      }
      event #15 {
        n205 = event-data() -> ()  [unwired: 2 out]
        n206 = local read "Target Pattern"() -> (w447:T15)
        n207 = local read "Mixed Mode Status"() -> (w446:T2)
        n208 = case shown="\"Reset Targets to Zero\"" w447 {
          tunnel: w452 -> [w456 w463]
          tunnel: [w456 w457] -> w444
          tunnel: w443 -> [w455 w460]
          tunnel: w442 -> [w454 w461]
          tunnel: [w455 w459] -> w441
          tunnel: [w454 w458] -> w440
          frame #0 {
          }
          frame #1 {
            n209 = Bundle By Name(cluster=w463, "Targets Updated"=TRUE) -> (w457:T9)
            n210 = Enqueue Element(queue=w461, element=w457, error in (no error)=w460) -> (queue out=w458:refnum<queue>, error out=w459:errorcluster)  [unwired: 2 out]
          }
        }
        n211 = call "Apply Target Pattern.vi"("Mixed Mode Status"=w446, "Target Pattern"=w447) -> ("Targets"=w449:T19[])  [unwired: 9 out]
        n212 = call "Step DAO.vi"("Step In"=w449, "Step DAO Actions"=Step_DAO_Actions."Set") -> ("Step Out"=w445:T19[])  [unwired: 2 in, 7 out]
        n213 = local write "Targets"(w445) -> ()
      }
      event #16 {
        n214 = event-data() -> ("NewVal"=w465:bool)  [unwired: 1 out]
        n215 = flat-sequence {
          tunnel: w465 -> [w473]
          tunnel: [w473] -> w464
          frame #0 {
            n216 = local write "Connect Server Flag"(w473) -> ()
          }
        }
        n217 = call "App Status Globals.vi"("App Status Actions"=App_Status_Actions."Set NTCP Link", "Status\nSetting"=w464) -> ()  [unwired: 12 in, 2 out]
      }
      event #17 {
        n218 = event-data() -> ("NewVal"=w482:bool)  [unwired: 1 out]
        n219 = Bundle By Name(cluster=w483, "Auto-Accept Enabled"=w482) -> (w477:T9)
        n220 = Enqueue Element(queue=w478, element=w477, error in (no error)=w476) -> (queue out=w474:refnum<queue>, error out=w475:errorcluster)  [unwired: 2 out]
      }
    }
    n221 = local read "App Running"() -> (w146:bool)
    n222 = Not(x=w146) -> (.not. x?=w142:bool)
    n223 = call "Error Logger.vi"("error in (no error)"=w154) -> ("error out"=w153:errorcluster)  [unwired: 1 in, 9 out]
  }
  n224 = call "NoArgumentsLauncher.vi"("error in (no error)"=w33, "Application"=NoPanelAppTypes."Data Archiving", "Application Launcher Actions"=Launcher_Actions."Stop") -> ()  [unwired: 9 out]
  n225 = Obtain Queue(name (unnamed)="From NTCP", element data type=w45) -> (queue out=w46:refnum<queue>)  [unwired: 3 in, 2 out]
  n226 = while {
    shift-right: [w499] -> _
    shift-left: NTCP_States."Init" ("NTCP State") -> [w500]
    shift-right: [w498] -> _
    shift-left: w44 -> [w497]
    shift-right: [w496] -> _
    shift-left: w45 -> [w495]
    shift-right: [w491] -> _
    shift-left: w22 -> [w490]
    shift-right: [w494] -> _
    shift-left: w46 -> [w493]
    shift-right: [w485] -> _
    shift-left: T19[] [] ("Step Out") -> [w486]
    tunnel: [w484] -> w14
    stop <- w484 stop-if-true
    # "NTCP Loop"
    n227 = local read "NTCP MM Requests"() -> (w488:T1)
    n228 = case shown="\"Shutdown Server\"" w500 {
      tunnel: [NTCP_States."Disconnected" ("NTCP State") w519 NTCP_States."Connect to Server" ("NTCP State") NTCP_States."Listening" ("NTCP State") w568 w581 NTCP_States."Listening" ("NTCP State") NTCP_States."Listening" ("NTCP State") NTCP_States."Listening" ("NTCP State") NTCP_States."Disconnected" ("NTCP State")] -> w499
      tunnel: [w509 w515 w531 w540 w558 w579 w627 w668 w702 w722] -> w498
      tunnel: w497 -> [w509 w515 w531 w540 w558 w580 w628 w668 w702 w722]
      tunnel: [w508 w514 w530 w542 w547 w576 w624 w670 w697 w724] -> w496
      tunnel: w495 -> [w508 w514 w530 w542 _ w576 w624 w670 w697 w724]
      tunnel: w490 -> [w503 w513 w523 w539 w560 w578 w626 w672 w693 w720]
      tunnel: [w502 w513 w526 w539 w561 w578 w626 w672 w691 w713] -> w492
      tunnel: [w504 w512 w529 w541 w562 w577 w625 w671 w701 w715] -> w494
      tunnel: w493 -> [w507 w512 w529 w541 w563 w577 w625 w671 w701 w721]
      tunnel: w488 -> [_ _ _ w535 _ _ _ w666 w703 w711]
      tunnel: [u32 200 ("millisecond multiple") u32 200 ("millisecond multiple") u32 10 ("millisecond multiple") u32 10 ("millisecond multiple") u32 10 ("millisecond multiple") u32 10 ("millisecond multiple") u32 10 ("millisecond multiple") u32 10 ("millisecond multiple") u32 10 ("millisecond multiple") u32 10 ("millisecond multiple")] -> w487
      tunnel: w486 -> [_ w510 w524 w536 w543 w571 w620 w664 w695 w712]
      tunnel: [T19[] [] ("Step Out") w510 w524 w536 w543 w571 w620 w662 T19[] [] ("Step Out") w712] -> w485
      frame #0 {
        n229 = Flush Queue(queue=w507, error in (no error)=w503) -> (queue out=w504:refnum<queue>, error out=w502:errorcluster)  [unwired: 1 out]
      }
      frame #1 {
        n230 = local read "Connect Server Flag"() -> (w517:bool)
        n231 = Select(t=NTCP_States."Start Server" ("NTCP State"), s=w517, f=NTCP_States."Disconnected" ("NTCP State")) -> (s? t:f=w519:T16)
      }
      frame #2 {
        n232 = call "App Status Globals.vi"("App Status Actions"=App_Status_Actions."Set NTCP Link", "Status\nSetting"=TRUE ("Status\nSetting"), "error in (no error)"=w523) -> ("error out"=w522:errorcluster)  [unwired: 11 in, 1 out]
        n233 = call "NoArgumentsLauncher.vi"("error in (no error)"=w522, "Application"=NoPanelAppTypes."NTCP Socket", "Application Launcher Actions"=Launcher_Actions."Launch") -> ("error out"=w526:errorcluster)  [unwired: 8 out]
      }
      frame #3 {
        w533 = TRUE ("Connected")
        n234 = Bundle By Name(cluster=w535, "Connected"=w533) -> (w534:T1)
        n235 = local write "Connected"(w533) -> ()
        n236 = local write "NTCP MM Requests"(w534) -> ()
      }
      frame #4 {
        n237 = local read "Connect Server Flag"() -> (w557:bool)
        n238 = Dequeue Element(queue=w563, timeout in ms (-1)=200, error in (no error)=w560) -> (queue out=w562:refnum<queue>, element=w547:T27, timed out?=w548:bool, error out=w561:errorcluster)
        n239 = Unbundle By Name(w547) -> ("NTCP commands"=w545:T28, "Payload"=w546:T29[])
        n240 = Index Array(array=w546, index=0) -> (element=w551:T29)
        n241 = Equal?(x=w545, y=NTCP_Commands."propose" ("NTCP commands")) -> (x = y?=w554:bool)
        n242 = Unbundle By Name(w551) -> ("Content"=w552:string)
        n243 = Empty String/Path?(string/path=w552) -> (empty?=w553:bool)
        n244 = Select(t=NTCP_States."Listening" ("NTCP State"), s=w557, f=NTCP_States."Shutdown Server") -> (s? t:f=w566:T16)
        n245 = Not(x=w548) -> (.not. x?=w544:bool)
        n246 = Compound Arithmetic op=AND(w544, w553, w554) -> (w555:bool)
        n247 = case shown="True" w555 {
          tunnel: [_ w569] -> _
          frame #0 {
          }
          frame #1 {
            n248 = One Button Dialog(message="AHA TOO!!!!!!!!!!!!") -> (true=w569:bool)  [unwired: 1 out]
          }
        }
        n249 = Select(t=NTCP_States."Parse Message" ("NTCP State"), s=w544, f=w566) -> (s? t:f=w568:T16)
      }
      frame #5 {
        n250 = Unbundle By Name(w576) -> ("NTCP commands"=w572:T28, "Transaction ID"=w575:string, "Payload"=w573:T29[])
        n251 = case shown="\"execute\"" w572 {
          tunnel: [NTCP_States."Proposed" ("NTCP State") NTCP_States."Execute" ("NTCP State") NTCP_States."Listening" ("NTCP State") NTCP_States."Listening" ("NTCP State") NTCP_States."Listening" ("NTCP State") NTCP_States."Listening" ("NTCP State") NTCP_States."Shutdown Server" ("NTCP State") NTCP_States."Shutdown Server" ("NTCP State") NTCP_States."Get Control Point" ("NTCP State") NTCP_States."Listening" ("NTCP State")] -> w581
          tunnel: w580 -> [w582 w587 w589 w591 w593 w595 w597 w599 w601 w607]
          tunnel: [w582 w587 w589 w591 w593 w595 w597 w599 w601 w607] -> w579
          tunnel: w573 -> [_ _ _ _ _ _ _ _ _ w606]
          tunnel: w575 -> [_ w584 _ _ _ _ _ _ _ _]
          frame #0 {
          }
          frame #1 {
            n252 = local read "Test Statistics"() -> (w585:cluster{"Steps":string, "Elapsed \nTime":dbl})
            n253 = Bundle By Name(cluster=w585, "Steps"=w584) -> (w586:cluster{"Steps":string, "Elapsed \nTime":dbl})
            n254 = local write "Test Statistics"(w586) -> ()
          }
          frame #2 {
          }
          frame #3 {
          }
          frame #4 {
          }
          frame #5 {
          }
          frame #6 {
          }
          frame #7 {
          }
          frame #8 {
          }
          frame #9 {
            n255 = Index Array(array=w606, index=0) -> (element=w604:T29)
            n256 = Unbundle By Name(w604) -> ("Content"=w603:string)
            n257 = Concatenate Strings("Message \"" ("string"), w603, "\" unknown" ("string")) -> (w610:string)
            n258 = One Button Dialog(message=w610) -> ()  [unwired: 2 out]
          }
        }
      }
      frame #6 {
        n259 = Unbundle By Name(w624) -> ("Payload"=w621:T29[], "Control Point"=w623:string)
        n260 = call "App Status Globals.vi"("App Status Actions"=App_Status_Actions."Get Status") -> ("App Status Out"=w613:T35)  [unwired: 5 in, 9 out]
        n261 = Unbundle By Name(w613) -> ("Cartesian Type"=w612:bool)
        n262 = Index Array(array=w621, index=0) -> (element=w616:T29)
        n263 = Unbundle By Name(w616) -> ("Control Point Suffix"=w615:T30)
        n264 = case shown="\"LBCB2\"" w615 {
          tunnel: [w630 w643 w656] -> w618
          tunnel: w612 -> [w634 w647 w659]
          frame #0 {
            n265 = call "Cartesian Data Set.vi"("Measurement Actions"=Cartesian_Measurment_Actions."Get", "LBCB Selected"=LBCB_Number."LBCB2") -> ("Cartesian Data Offsets Out"=w635:T49, "Cartesian Data Hold Data Out"=w640:T49)  [unwired: 4 in, 8 out]
            n266 = Unbundle By Name(w640) -> ("Displacements"=w639:dbl[], "Forces"=w638:dbl[])
            n267 = Unbundle By Name(w635) -> ("Displacements"=w636:dbl[], "Forces"=w637:dbl[])
            n268 = Build Array (concatenate)(w639, w638) -> (w631:dbl[])
            n269 = Build Array (concatenate)(w636, w637) -> (w632:dbl[])
            n270 = call "Shift Cartesian Axes.vi"("Coordianate Offset"=w632, "Coordinate Switch"=w634, "Coordianate Input"=w631, "Direction"=enum16{" +", " - "}." - ") -> ("Coordianate Output"=w630:dbl[])
          }
          frame #1 {
            n271 = call "Cartesian Data Set.vi"("Measurement Actions"=Cartesian_Measurment_Actions."Get", "LBCB Selected"=LBCB_Number."LBCB1") -> ("Cartesian Data Offsets Out"=w648:T49, "Cartesian Data Hold Data Out"=w653:T49)  [unwired: 4 in, 8 out]
            n272 = Unbundle By Name(w653) -> ("Displacements"=w652:dbl[], "Forces"=w651:dbl[])
            n273 = Unbundle By Name(w648) -> ("Displacements"=w649:dbl[], "Forces"=w650:dbl[])
            n274 = Build Array (concatenate)(w652, w651) -> (w644:dbl[])
            n275 = Build Array (concatenate)(w649, w650) -> (w645:dbl[])
            n276 = call "Shift Cartesian Axes.vi"("Coordianate Offset"=w645, "Coordinate Switch"=w647, "Coordianate Input"=w644, "Direction"=enum16{" +", " - "}." - ") -> ("Coordianate Output"=w643:dbl[])
          }
          frame #2 {
            n277 = call "External Sensors Data Set.vi"("Measurement Actions"=Cartesian_Measurment_Actions."Get") -> ("Offsets"=w657:dbl[], "Hold Data Out"=w658:dbl[])  [unwired: 3 in, 6 out]
            n278 = call "Shift Cartesian Axes.vi"("Coordianate Offset"=w657, "Coordinate Switch"=w659, "Coordianate Input"=w658, "Direction"=enum16{" +", " - "}." - ") -> ("Coordianate Output"=w656:dbl[])
          }
        }
        n279 = call "NTCP Send Msgs.vi"("Message Type"=NTCP_Msg_Types."Control Point", "queue in"=w628, "Hold Data"=w618, "Contol\nPoint\nSuffix"=w615, "ControlPoint name"=w623) -> ("queue out"=w627:refnum<queue>)  [unwired: 3 in, 7 out]
      }
      frame #7 {
        n280 = Unbundle By Name(w670) -> ("Payload"=w665:T29[])
        n281 = for {
          shift-right: [w681] -> w663
          shift-left: w664 -> [w682]
          tunnel: w665 -> [w680] mode=indexing
          n282 = Unbundle By Name(w680) -> ("Content"=w677:string, "Control Point Suffix"=w679:T30)
          n283 = Empty String/Path?(string/path=w677) -> (empty?=w678:bool)
          n284 = case shown="True" w678 {
            tunnel: w682 -> [w688 w690]
            tunnel: [w685 w690] -> w681
            tunnel: w679 -> [w684 _]
            tunnel: w677 -> [w683 _]
            frame #0 {
              n285 = call "ntcp command.vi"("Input string"=w683) -> ("NTCP Command"=w689:T50)  [unwired: 1 in, 1 out]
              n286 = call "NTCP Command 2 Targets.vi"("NTCP Command"=w689, "Targets In"=w688, "Contol\nPoint\nSuffix"=w684) -> ("Targets Out"=w686:T19[])  [unwired: 8 out]
              n287 = call "Step DAO.vi"("Step In"=w686, "Step DAO Actions"=Step_DAO_Actions."Set") -> ("Step Out"=w685:T19[])  [unwired: 2 in, 7 out]
            }
            frame #1 {
            }
          }
        }
        n288 = flat-sequence {
          tunnel: w666 -> [w676]
          tunnel: w663 -> [w673]
          tunnel: [w673] -> w662
          frame #0 {
            n289 = Bundle By Name(cluster=w676, "Propose Pending"=TRUE) -> (w675:T1)
            n290 = local write "NTCP MM Requests"(w675) -> ()
          }
        }
      }
      frame #8 {
        n291 = Unbundle By Name(w697) -> ("Transaction ID"=w696:string)
        n292 = call "Step DAO.vi"("error in (no error)"=w693, "Step Count In"=w696, "Step In"=w695, "Step DAO Actions"=Step_DAO_Actions."Set") -> ("error out"=w692:errorcluster)  [unwired: 7 out]
        n293 = flat-sequence {
          tunnel: w703 -> [w707]
          tunnel: w692 -> [w704]
          tunnel: [w704] -> w691
          frame #0 {
            n294 = Bundle By Name(cluster=w707, "Execute Pending"=TRUE ("Start Requested")) -> (w706:T1)
            n295 = local write "NTCP MM Requests"(w706) -> ()
          }
        }
      }
      frame #9 {
        w709 = FALSE ("Execute Pending")
        w716 = FALSE ("Connect")
        n296 = local write "Connected"(w716) -> ()
        n297 = Bundle By Name(cluster=w711, "Connected"=w709) -> (w710:T1)
        n298 = call "App Status Globals.vi"("App Status Actions"=App_Status_Actions."Set NTCP Link", "Status\nSetting"=w709) -> ()  [unwired: 12 in, 2 out]
        n299 = call "NoArgumentsLauncher.vi"("error in (no error)"=w720, "Application"=NoPanelAppTypes."NTCP Socket", "Application Launcher Actions"=Launcher_Actions."Stop") -> ("error out"=w714:errorcluster)  [unwired: 8 out]
        n300 = Flush Queue(queue=w721, error in (no error)=w714) -> (queue out=w715:refnum<queue>, error out=w713:errorcluster)  [unwired: 1 out]
        n301 = local write "Connect Server Flag"(w716) -> ()
        n302 = local write "Connect Server"(w716) -> ()
        n303 = local write "NTCP MM Requests"(w710) -> ()
      }
    }
    n304 = Wait Until Next ms Multiple(millisecond multiple=w487) -> ()  [unwired: 1 out]
    n305 = local read "App Running"() -> (w489:bool)
    n306 = call "Error Logger.vi"("error in (no error)"=w492) -> ("error out"=w491:errorcluster)  [unwired: 1 in, 9 out]
    n307 = Not(x=w489) -> (.not. x?=w484:bool)
    "NTCP State" <- w500
  }
  n308 = Multiply(x=6.0, y=3600.0) -> (x*y=w37:dbl)
  n309 = while {
    shift-right: [w781] -> _
    shift-left: w23 -> [w782]
    shift-right: [w777] -> _
    shift-left: w40 -> [w778]
    shift-right: [w780] -> _
    shift-left: w19 -> [w759]
    shift-right: [w775] -> _
    shift-left: Mixed_Mode_Widget_State."Idle" ("Mixed Mode Widget Action Buttons") -> [w751]
    shift-right: [w744] -> _
    shift-left: w21 -> [w743]
    shift-right: [w764] -> _
    shift-left: w44 -> [w765]
    tunnel: w37 -> [_]
    shift-right: [w766] -> _
    shift-left: _ -> [w774]
    shift-right: [w740] -> _
    shift-left: w18 -> [w742]
    tunnel: [w729] -> w15
    shift-right: [w736] -> _
    shift-left: w6 -> [w738]
    shift-right: [w726] -> _
    shift-left: _ -> [w733]
    stop <- w729 stop-if-true
    # "Mixed Mode State Machine"
    n310 = case shown="\"Exit\"" w751 {
      tunnel: [FALSE TRUE FALSE FALSE FALSE FALSE FALSE FALSE FALSE FALSE] -> w749
      frame #0 {
      }
      frame #1 {
      }
      frame #2 {
      }
      frame #3 {
      }
      frame #4 {
      }
      frame #5 {
      }
      frame #6 {
      }
      frame #7 {
      }
      frame #8 {
      }
      frame #9 {
      }
    }
    n311 = Wait on Notification(notifier=w782, timeout in ms (-1)=50, error in (no error)=w759) -> (notifier out=w781:refnum<notifier>, notification=w746:T5, timed out?=w745:bool, error out=w732:errorcluster)  [unwired: 1 out]
    n312 = Dequeue Element(queue=w738, timeout in ms (-1)=u32 300 ("millisecond multiple"), error in (no error)=w732) -> (queue out=w736:refnum<queue>, element=w735:T9, timed out?=w734:bool, error out=w731:errorcluster)
    n313 = local read "NTCP MM Requests"() -> (w763:T1)
    n314 = Select(t=w733, s=w734, f=w735) -> (s? t:f=w728:T9)
    n315 = call "Fault List 2 Indicators.vi"() -> ("Forces"=w758:bool, "Displacement"=w757:bool)  [unwired: 1 in, 9 out]
    n316 = Unbundle By Name(w728) -> ("Stop Requested"=w753:bool, "Exit Requested"=w752:bool)
    n317 = case shown="False" w745 {
      tunnel: w746 -> [w785 _]
      tunnel: [w785 w786] -> w744
      tunnel: w743 -> [_ w786]
      frame #0 {
        n318 = call "States 2 Leds.vi"("MixedModeStates"=w785) -> ("Mixed Mode State Display"=w784:T18)  [unwired: 10 out]
        n319 = local write "Mixed Mode State Display"(w784) -> ()
      }
      frame #1 {
      }
    }
    n320 = Compound Arithmetic op=OR(w753, w757, w758) -> (w755:bool)
    n321 = And(x=w749, y=w755) -> (x .and. y?=w750:bool)
    n322 = Select(t=Mixed_Mode_Widget_State."Exit", s=w752, f=w751) -> (s? t:f=w760:T8)
    n323 = Select(t=Mixed_Mode_Widget_State."Limit Fault", s=w750, f=w760) -> (s? t:f=w756:T8)
    n324 = local read "Mixed Mode Command"() -> (w776:T11)
    n325 = case shown="\"Manual\"" "Mixed Mode Control Type" {
      tunnel: w756 -> [w828 w835 w849]
      tunnel: w728 -> [w829 w839 w851]
      tunnel: w774 -> [w827 w834 w847]
      tunnel: [w826 w837 w846] -> w725
      tunnel: w778 -> [w825 w841 w856]
      tunnel: [w824 w833 w854] -> w777
      tunnel: w744 -> [w823 w832 w842]
      tunnel: w776 -> [w822 w840 w852]
      tunnel: [w821 w836 w848] -> w775
      tunnel: [w820 w838 w850] -> w727
      tunnel: w765 -> [w819 w831 w855]
      tunnel: [w819 w831 w853] -> w764
      tunnel: w763 -> [w818 w830 w844]
      tunnel: [w818 w830 w843] -> w748
      frame #0 {
        n326 = call "Manual Mode State Machine.vi"("Mixed Mode Command In"=w822, "MM In"=w825, "MixedModeStates In"=w823, "Mixed Mode Blinkies In"=w827, "Mixed Mode Widget Actions In"=w828, "Mixed Mode Widget Requests"=w829) -> ("Mixed Mode Blinkies Out"=w826:T51, "Mixed Mode Widget Actions Out"=w821:T8, "Mixed Mode Widget Approval"=w820:T44, "MM Out"=w824:refnum<queue>)  [unwired: 2 out]
      }
      frame #1 {
        n327 = call "Input File Mode State Machine.vi"("Mixed Mode Widget Requests"=w839, "MM In"=w841, "Mixed Mode Command In"=w840, "Mixed Mode Widget Actions In"=w835, "Mixed Mode Blinkies In"=w834, "MixedModeStates In"=w832) -> ("Mixed Mode Widget Approval"=w838:T9, "Mixed Mode Widget Actions Out"=w836:T8, "Mixed Mode Blinkies Out"=w837:T51, "MM Out"=w833:refnum<queue>)  [unwired: 6 out]
      }
      frame #2 {
        n328 = local read "Control Point"() -> (w845:string)
        n329 = call "NTCP Mode State Machine.vi"("Mixed Mode Widget Requests"=w851, "MM In"=w856, "Mixed Mode Command In"=w852, "NTCP In"=w855, "Mixed Mode Widget Actions In"=w849, "Mixed Mode Blinkies In"=w847, "NTCP MM Requests In"=w844, "ControlPoint name"=w845, "MixedModeStates In"=w842) -> ("Mixed Mode Widget Approval"=w850:T9, "Mixed Mode Widget Actions Out"=w848:T8, "Mixed Mode Blinkies Out"=w846:T51, "NTCP MM Requests Out"=w843:T1, "MM Out"=w854:refnum<queue>, "NTCP Out"=w853:refnum<queue>)  [unwired: 1 out]
      }
    }
    "Mixed Mode Widget Actions" <- w775
    n330 = local read "App Running"() -> (w730:bool)
    n331 = Not(x=w730) -> (.not. x?=w729:bool)
    n332 = Unbundle By Name(w748) -> ("Reset"=w747:bool)
    n333 = Unbundle By Name(w727) -> ("Reset"=w762:bool, "Running"=w739:bool)
    n334 = Unbundle By Name(w725) -> ("Blink Accept"=w772:bool, "Blink Start"=w768:bool, "Targets Updated"=w767:bool)  [unwired: 1 out]
    n335 = Unbundle By Name(w774) -> ("Blink Accept"=w773:bool, "Blink Start"=w769:bool)
    n336 = case shown="True" w747 {
      tunnel: w748 -> [_ w789]
      frame #0 {
      }
      frame #1 {
        n337 = Bundle By Name(cluster=w789, "Reset"=FALSE) -> (w788:T1)
        n338 = local write "NTCP MM Requests"(w788) -> ()
      }
    }
    n339 = Exclusive Or(1:w772, 2:w773) -> (0:w771:bool)
    n340 = Exclusive Or(1:w768, 2:w769) -> (0:w770:bool)
    n341 = case shown="False" w771 {
      tunnel: w772 -> [_ w817]
      frame #0 {
      }
      frame #1 {
        n342 = property on="Accept" class="Bool (strict)"("Blinking"=w817) -> ()  [unwired: 2 in, 2 out]
      }
    }
    n343 = case shown="False" w770 {
      tunnel: w768 -> [_ w816]
      frame #0 {
      }
      frame #1 {
        n344 = property on="Start" class="Bool (strict)"("Blinking"=w816) -> ()  [unwired: 2 in, 2 out]
      }
    }
    n345 = case shown="True" w762 {
      tunnel: w727 -> [w800 w803]
      tunnel: w739 -> [_ _]
      tunnel: w742 -> [w801 w809]
      tunnel: w731 -> [w802 w808]
      tunnel: [w802 w807] -> w741
      tunnel: [w801 w806] -> w740
      tunnel: [w800 w804] -> w726
      frame #0 {
      }
      frame #1 {
        n346 = Bundle By Name(cluster=w803, "Reset"=FALSE) -> (w804:T9)
        n347 = Enqueue Element(queue=w809, element=w803, error in (no error)=w808) -> (queue out=w806:refnum<queue>, error out=w807:errorcluster)  [unwired: 2 out]
      }
    }
    n348 = case shown="False" w767 {
      tunnel: w725 -> [w810 w813]
      tunnel: [w810 w811] -> w766
      frame #0 {
      }
      frame #1 {
        n349 = call "Step DAO.vi"("Step DAO Actions"=Step_DAO_Actions."Get") -> ("Step Out"=w814:T19[])  [unwired: 3 in, 7 out]
        n350 = Bundle By Name(cluster=w813, "Targets Updated"=FALSE) -> (w811:T51)
        n351 = local write "Targets"(w814) -> ()
      }
    }
    n352 = call "Error Logger.vi"("error in (no error)"=w741) -> ("error out"=w780:errorcluster)  [unwired: 1 in, 9 out]
  }
  n353 = Obtain Notifier(name (unnamed)="Mixed Mode Statuses", notification data type=T2 {"LBCB Target"=[], "MixedModeStates"=enum."Init", "LBCB Convergence"=[], "LBCB Measurements"=[]} ("Mixed Mode Status"), error in (no error)=w22) -> (notifier out=w27:refnum<notifier>, error out=w26:errorcluster)  [unwired: 1 in, 1 out]
  n354 = while {
    shift-right: [w862] -> _
    shift-left: w27 -> [w864]
    shift-right: [w861] -> _
    shift-left: w26 -> [w863]
    tunnel: [w857] -> w16
    stop <- w857 stop-if-true
    # "Mixed Mode Target Display"
    n355 = Wait on Notification(notifier=w864, timeout in ms (-1)=50, error in (no error)=w863) -> (notifier out=w862:refnum<notifier>, notification=w860:T2, timed out?=w858:bool, error out=w861:errorcluster)  [unwired: 1 out]
    n356 = case shown="False" w858 {
      tunnel: w860 -> [w866 _]
      frame #0 {
        n357 = Unbundle By Name(w866) -> ("LBCB 1 Measurements"=w870:T7, "LBCB 2 Measurements"=w869:T7)
        n358 = call "Measurements 2 Target Arrays.vi"(9:w869, "LBCB Command Data"=w870, "Target  Inputs"="Targets") -> ("Target  Outputs"=→"Current Values":T19[])  [unwired: 8 out]
        "Mixed Mode Status" <- w866
      }
      frame #1 {
      }
    }
    n359 = local read "App Running"() -> (w859:bool)
    n360 = Not(x=w859) -> (.not. x?=w857:bool)
  }
  n361 = Compound Arithmetic op=AND(w15, w12, w13, w14, w16) -> (w11:bool)
  n362 = Not(x=w11) -> (.not. x?=w4:bool)
  n363 = flat-sequence {
    tunnel: w4 -> [w873]
    tunnel: [w873] -> w3
    frame #0 {
      n364 = control-ref of="This VI"() -> (w872:refnum<vi>)
      n365 = property class="VI"(reference=w872, "Front Panel.Open"=FALSE ("Front Panel Window:Open")) -> ()  [unwired: 1 in, 2 out]
    }
  }
  n366 = local write "Stop"(w3) -> ()
